vi "Scope_5782_6channel_IQ_PID.vi"() -> ()   [LabVIEW 2018]
uses:
  FPGA/DataMode.ctl
  <vilib>/Analysis/4window.llb/windowTd.ctl
  Host/Scope/controls/power_spectrum_unit.ctl
  Host/Scope5782/Scope/controls/5782_trigger_type.ctl
  Host/Scope/controls/Data_calc_mode.ctl
  Host/Scope/controls/Data_display_mode.ctl
  Host/Scope/controls/Graph_references.ctl
  Host/Scope/controls/graph_controls.ctl
  Host/Scope/controls/Channel_select_2fpga.ctl
  <vilib>/userdefined/High Color/nirio_resource_hc.ctl
  Host/Scope/controls/All FP controls.ctl
  Host/Scope/controls/Output scale.ctl
  Host/Communication/Driver/RemoteConnection/RemoteReferences.ctl
  Host/FpgaRef/FpgaRef5761/ClockSource_5761.ctl
  Host/INI files/Settings file IQ PID/SettingsFileIQpid.lvclass
  C:/PXIe/InProgress/source/Host/INI files/Settings file base/SettingsFile.lvclass
  Host/Communication/Driver/RemoteConnection/RemoteConnection.lvclass
  Host/Scope/Scope5782_six_channel/Scope5782_six_channel.lvclass
  C:/PXIe/InProgress/source/Host/Scope/ScopeBase/ScopeBase.lvclass
  Host/Scope/ScopeBase/ScopeBase.lvclass/ScopeBase.ctl
  Host/INI files/Settings file base/Save event.ctl
  FPGA/fpga_settings.ctl
  Host/Scope/Scope5782_six_channel/Scope5782_six_channel.lvclass/Scope5782_six_channel.ctl
  Host/Scope/controls/ScopeMode.ctl
  Host/FpgaRef/FpgaRef5761/FpgaRef5761.lvclass
  C:/PXIe/InProgress/source/Host/FpgaRef/FpgaRefBase/FpgaRefBase.lvclass
  Host/FpgaRef/FpgaRef5782/FpgaRef5782.lvclass
  Host/Communication/global_stop.vi
  <vilib>/FPGAPlugInAG/PXIe-7975R/niLvFpga_Open_PXIe-7975R.vi
  <vilib>/rvi/interface/common/dynamic/niFpgaDynamicAddResources.vi
  Host/Communication/response.ctl
  Host/Communication/driver_status.ctl
  <vilib>/rvi/interface/nirviOpenFPGA/nirviOpenFPGA.xnode
  FPGA Bitfiles/FPGAmain_5782_IQ_PID_PtIU9Q++q2U.lvbitx
  FPGA Bitfiles/FPGAmain_5761_zuew0qNtRjU.lvbitx
  <vilib>/rvi/FXPMathLib/FxpInterpret/XNode/nifxpmath_Interpret.xnode
  Host/Communication/Driver/TcpServerDriver/TcpServerDriver.lvclass
  Host/Scope/ScopeBase/ScopeBase.lvclass
  Host/INI files/Settings file base/SettingsFile.lvclass
  Host/FpgaRef/FpgaRefBase/FpgaRefBase.lvclass
  <vilib>/Analysis/NI_AALPro.lvlib
panel:
  out "All FP controls":T1
  in  "Show buffers":bool
  out "Adaptive FF graph":dbl[][](graph)
  in  "Tab Control":T2(tab)
  in  "Feedback I":bool caption="I Feedback"
  in  "Ki*T AM":fxp<+/-,32,4> caption="Ki*T"
  in  "Kd/T AM":fxp<+/-,32,4> caption="Kd/T"
  in  "Kp AM":fxp<+/-,32,4> caption="Kp"
  in  "Feedback delay":u32
  in  "Trigger delay":u32
  in  "Acquire samples":u32
  in  "Kp Q":fxp<+/-,32,4> caption="Kp"
  in  "Kd/T  Q":fxp<+/-,32,4> caption="Kd/T"
  in  "Ki*T Q":fxp<+/-,32,4> caption="Ki*T"
  in  "Feedback Q":bool caption="Q Feedback"
  in  "Host scale 5761":T3 caption="Host scale"
  in  "Input scale 5761":T3 caption="Input scale"
  in  "Host scale":T3
  in  "Input scale":T3
  in  "Output scale":T3
  in  "ch2 DC offset":dbl caption="DC offset\nChannel 2"
  in  "ch3 DC offset":dbl caption="DC offset\nChannel 3"
  in  "ch0 DC offset 2":dbl caption="DC offset\nChannel 0"
  in  "ch1 DC offset 2":dbl caption="DC offset\nChannel 1"
  in  "ch0 DC offset":dbl caption="DC offset\nChannel 0"
  in  "ch1 DC offset":dbl caption="DC offset\nChannel 1"
  in  "Setpoint":path
  in  "Beam":path
  in  "Feed forward":path
  in  "show setpoint":bool
  in  "show beam":bool
  in  "show feedforward":bool
  in  "Setpoint enabled":bool
  in  "Beam/FF enabled":bool
  in  "IIR filter cutoff fequency [MHz]":dbl min=0.0 max=10000.0
  in  "Save FF to file":bool
  in  "Clear buffers":bool
  in  "Samples to skip":i32 min=0 max=400000
  in  "Adaptation factor [0-1]":dbl min=0.0 max=1.0
  in  "LP filter cutoff fequency [MHz]":dbl min=0.0 max=10000.0
  in  "Adaptive FF enabled":bool
  in  "Read buffers":bool
  in  "Virtual cavity":bool
  in  "Cavity model":bool
  in  "w12":dbl format="%#_12g"
  in  "R1":dbl
  in  "w1":dbl
  in  "Q1":dbl
  in  "K1":dbl
  in  "S":dbl=0.001 min=0.001 max=1000.0 format="%#_12g"
  in  "Input delay 5785":u32
  in  "Input delay 5761":u32
  in  "5761 resource":T4="PXI2Slot11"
  in  "5782 resource":T4="PXI2Slot18"
  in  "High speed transfer to host":bool=TRUE
  in  "Output enabled":bool=TRUE
  in  "Output delay delta":dbl(slide) scale=0.0..6.0
  in  "Output delay":dbl(slide) scale=0.0..6.0
  in  "Output mixer fequency [MHz]":dbl
  in  "Trigger":T5
  in  "Mode":T6
  in  "Mixer freq [MHz]":dbl
  in  "Unwrap phase":bool
  in  "#bins":i32=1 min=1 max=16
  in  "Unit":T7
  in  "Window":T8=1 items=["Rectangle"=0, "Hanning"=1, "Hamming"=2, "Blackman-Harris"=3, "Exact Blackman"=4, "Blackman"=5, "Flat Top"=6, "4 Term B-Harris "=7, "7 Term B-Harris"=8, "Low Sidelobe"=9, "Blackman Nuttall"=11, "Triangle"=30, "Bartlett-Hanning"=31, "Bohman"=32, "Parzen"=33, "Welch"=34, "Kaiser"=60, "Dolph-Chebyshev"=61, "Gaussian"=62]
  in  "Chart length":i32=400000
  in  "Trigmode":enum32{"Triggered", "Continuous"}(radio)
  in  "Reference for phase":T9
  in  "Graph_refs":T10
  out "Lower chart":dbl[][](graph)
  out "Upper chart":dbl[][](graph)
  out "Lower graph":i16[][](graph)
  in  "Buffer":T12
  in  "Display":T13
  out "stop 2":bool
  in  "Zoom freq X":bool
  in  "Zoom freq Y":bool
  in  "Zoom time Y":bool
  in  "Zoom time X":bool
  in  "Samples per 5782 record":i32
  in  "Phase offset (deg)":dbl
  in  "Fequency [MHz]":dbl format="%#_8g"
  out "freqdata":cluster{"f0":dbl, "df":dbl, "magnitude":dbl[]}[](graph)
  out "Upper graph":i16[][](graph)
  in  "Rumode":bool
  in  "Singleshot":bool
  out "error IO":errorcluster
  in  "stop":bool
  # "FPGA setup"
  # "ns"
  # "Output delay"
  # "Auto Zoom"
  # "FFT"
  # "Auto Zoom"
  # "Delays"
  # "5785"
  # "5761"
  # "5782"
  # "V"
  # "V"
  # "5761"
  # "V"
  # "V"
  # "V"
  # "V"
  # "Simulated data"
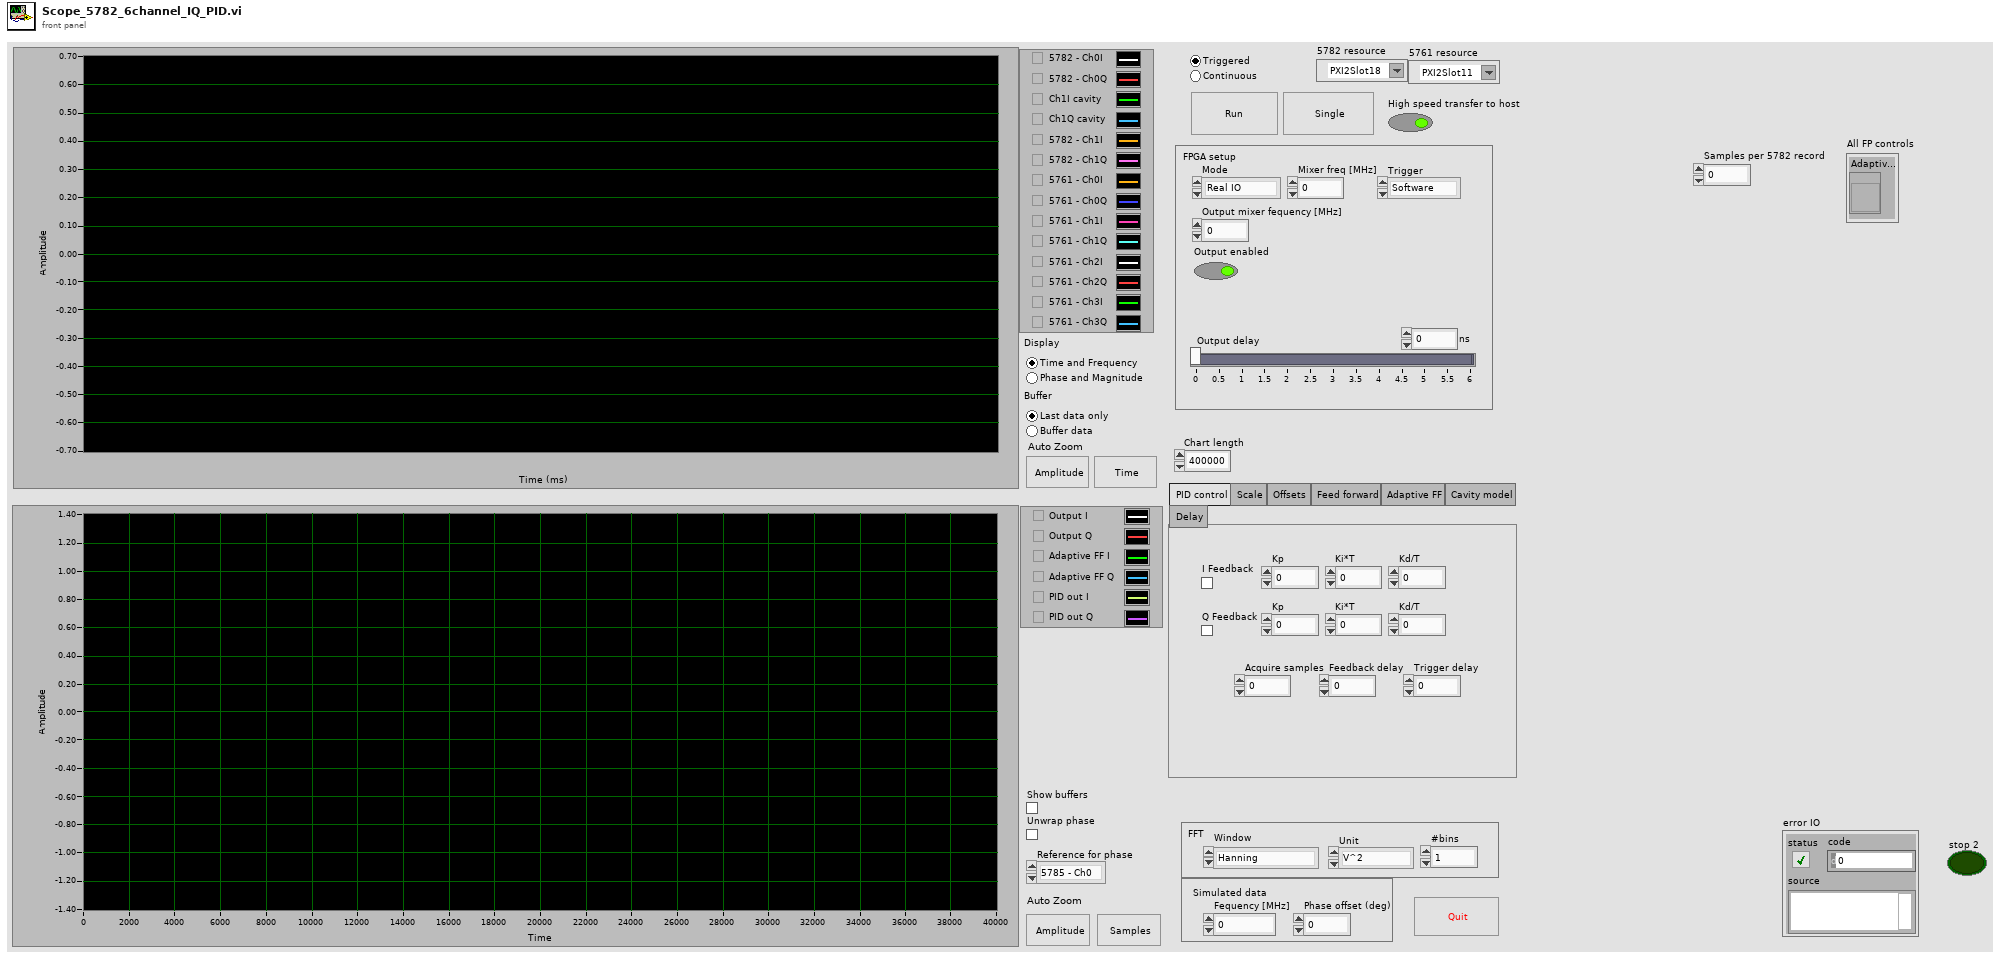
[diagram p1: front panel]
types:
  T1 = typedef "All FP controls.ctl" = cluster{"Adaptive FF enabled":refnum<vi>, "LP filter cutoff fequency [MHz]":refnum<vi>, "Adaptation factor [0-1]":refnum<vi>, "Samples to skip":refnum<vi>, "ch1 DC offset":refnum<vi>, "ch0 DC offset":refnum<vi>, "ch1 DC offset 2":refnum<vi>, "ch0 DC offset 2":refnum<vi>, "ch3 DC offset":refnum<vi>, "ch2 DC offset":refnum<vi>, "Feedback Q":refnum<vi>, "Ki*T Q":refnum<vi>, "Kd/T  Q":refnum<vi>, "Kp Q":refnum<vi>, "Acquire samples":refnum<vi>, "Trigger delay":refnum<vi>, "Feedback delay":refnum<vi>, "Kp AM":refnum<vi>, "Kd/T AM":refnum<vi>, "Ki*T AM":refnum<vi>, "Feedback I":refnum<vi>, "#bins":refnum<vi>, "Window":refnum<vi>, "Unit":refnum<vi>, "Input delay 5761":refnum<vi>, "Input delay 5785":refnum<vi>, "S":refnum<vi>, "K1":refnum<vi>, "Q1":refnum<vi>, "R1":refnum<vi>, "w12":refnum<vi>, "Cavity model":refnum<vi>, "w1":refnum<vi>, "Mode":refnum<vi>, "Trigger":refnum<vi>, "Output mixer fequency [MHz]":refnum<vi>, "Output delay":refnum<vi>, "Mixer freq [MHz]":refnum<vi>, "Triggered":refnum<vi>, "High speed transfer to host":refnum<vi>, "Continuous":refnum<vi>, "Output scale":refnum<vi>, "Host scale":refnum<vi>, "Input scale":refnum<vi>, "IIR filter cutoff fequency [MHz]":refnum<vi>, "Host scale 5761":refnum<vi>, "Virtual cavity":refnum<vi>, "Input scale 5761":refnum<vi>}
  T2 = enum32{"PID control", "Scale", "Offsets", "Feed forward", "Adaptive FF", "Cavity model", "Delay"}
  T3 = typedef "Output scale.ctl" = enum16{"x1", "x2", "x4", "x8", "x16", "x32"}
  T4 = typedef "nirio_resource_hc.ctl" = tag
  T5 = typedef "5782_trigger_type.ctl" = enum16{"Software", "Trigger input"}
  T6 = typedef "DataMode.ctl" = enum16{"Real IO", "Simulated"}
  T7 = typedef "power_spectrum_unit.ctl" = enum16{"V^2", "V", "dBV"}
  T8 = typedef "NI_AALPro.lvlib/windowTd.ctl" = u32
  T9 = typedef "Channel_select_2fpga.ctl" = enum16{"5785 - Ch0", "5785 - Ch1 cavity", "5785 - Ch1", "5761 - Ch0", "5761 - Ch1", "5761 - Ch2", "5761 - Ch3"}
  T10 = typedef "Graph_references.ctl" = cluster{"upper":T11, "lower":T11, "Freq graph":refnum<vi>, "Adaptive FF graph":refnum<vi>}
  T11 = typedef "graph_controls.ctl" = cluster{"Graph":refnum<vi>, "Time btn":refnum<vi>, "Amplitude btn":refnum<vi>, "Chart":refnum<vi>}
  T12 = typedef "Data_display_mode.ctl" = enum32{"Last data only", "Buffer data"}
  T13 = typedef "Data_calc_mode.ctl" = enum32{"Time and Frequency", "Phase and Magnitude"}
  T14 = typedef "ClockSource_5761.ctl" = enum8{"Internal Clock PLL Off", "Internal Clock PLL On (CLK_IN)", "External Clock (CLK_IN)", "Internal Clock PLL On (IoModSyncClk)", "External Clock (IoModSyncClk)"}
  T15 = typedef "RemoteConnection.lvclass/RemoteReferences.ctl" = cluster{"a":refnum<vi>, "b":refnum<vi>, "fm":refnum<vi>, "Output delay":refnum<vi>, "Output delay delta":refnum<vi>}
  T16 = typedef "response.ctl" = cluster{"driver status":T17, "Sender":string, "Type":i32, "Variant":variant}
  T17 = typedef "driver_status.ctl" = enum16{"Normal", "Startup", "Connection lost", "Reconnected", "Timeout", "Idle", "Busy"}
  T18 = typedef "message_queue.ctl" = refnum<queue>
  T19 = enum8{"Internal Clock PLL Off", "Internal Clock PLL On (REF IN)", "External Clock (CLK_IN)", "Internal Clock PLL On (IoModSyncClk)"}
  T20 = typedef "INI Save Event.ctl" = refnum<user-event>
  T21 = typedef "Save event.ctl" = cluster{"Automatic":bool, "Save":bool}
  T22 = typedef "fpga_settings.ctl" = enum16{"Feedback Enable", "New FIR coeffs", "FIR shift", "Enable filter", "Set Downsample", "Downsample", "CIC Gain", "Record length", "Trigger samples", "Quiet time", "a_am", "b_am", "Use fixed delay", "fixed sin_fi", "fixed cos_fi", "Ki*Tau", "Kp", "Kd_Tau", "Fi_start", "Fi_delta", "DC_offs 0", "DC_offs 1", "DC_offs 2", "DC_offs 3", "Ki*Tau am", "Kp am", "Kd_Tau am", "Feedback AM", "Trigger delay", "Feedback delay", "Setpoint enable", "Beam enable", "Samples to acquire", "Cavity Enable", "Cavity C1", "Cavity C2", "Cavity C3", "Cavity C4", "Cavity C5", "Input delay", "Ki*Tau Q", "Kp Q", "Kd_Tau Q", "Adaptive FF enable", "Feedforward a0", "Feedforward b0", "FF src adress", "FF dest adress", "Output scale", "Input scale", "Host scale", "FF_IIR b0", "FF_IIR b1", "FF_IIR b2", "FF_IIR-a1", "FF_IIR-a2", "Enable HW trigger", "Virtual cavity"}
  T23 = typedef "ScopeMode.ctl" = enum16{"Stopped", "Single", "Running", "Continuous"}
  T24 = enum8{"Enabled", "Disabled", "Disabled and Grayed Out"}
  T25 = typedef "Feedforward.ctl" = cluster{"Beam I":dbl[], "Beam Q":dbl[], "Feedforward I":dbl[], "Feedforward Q":dbl[], "Setpoint I":dbl[], "Setpoint Q":dbl[]}
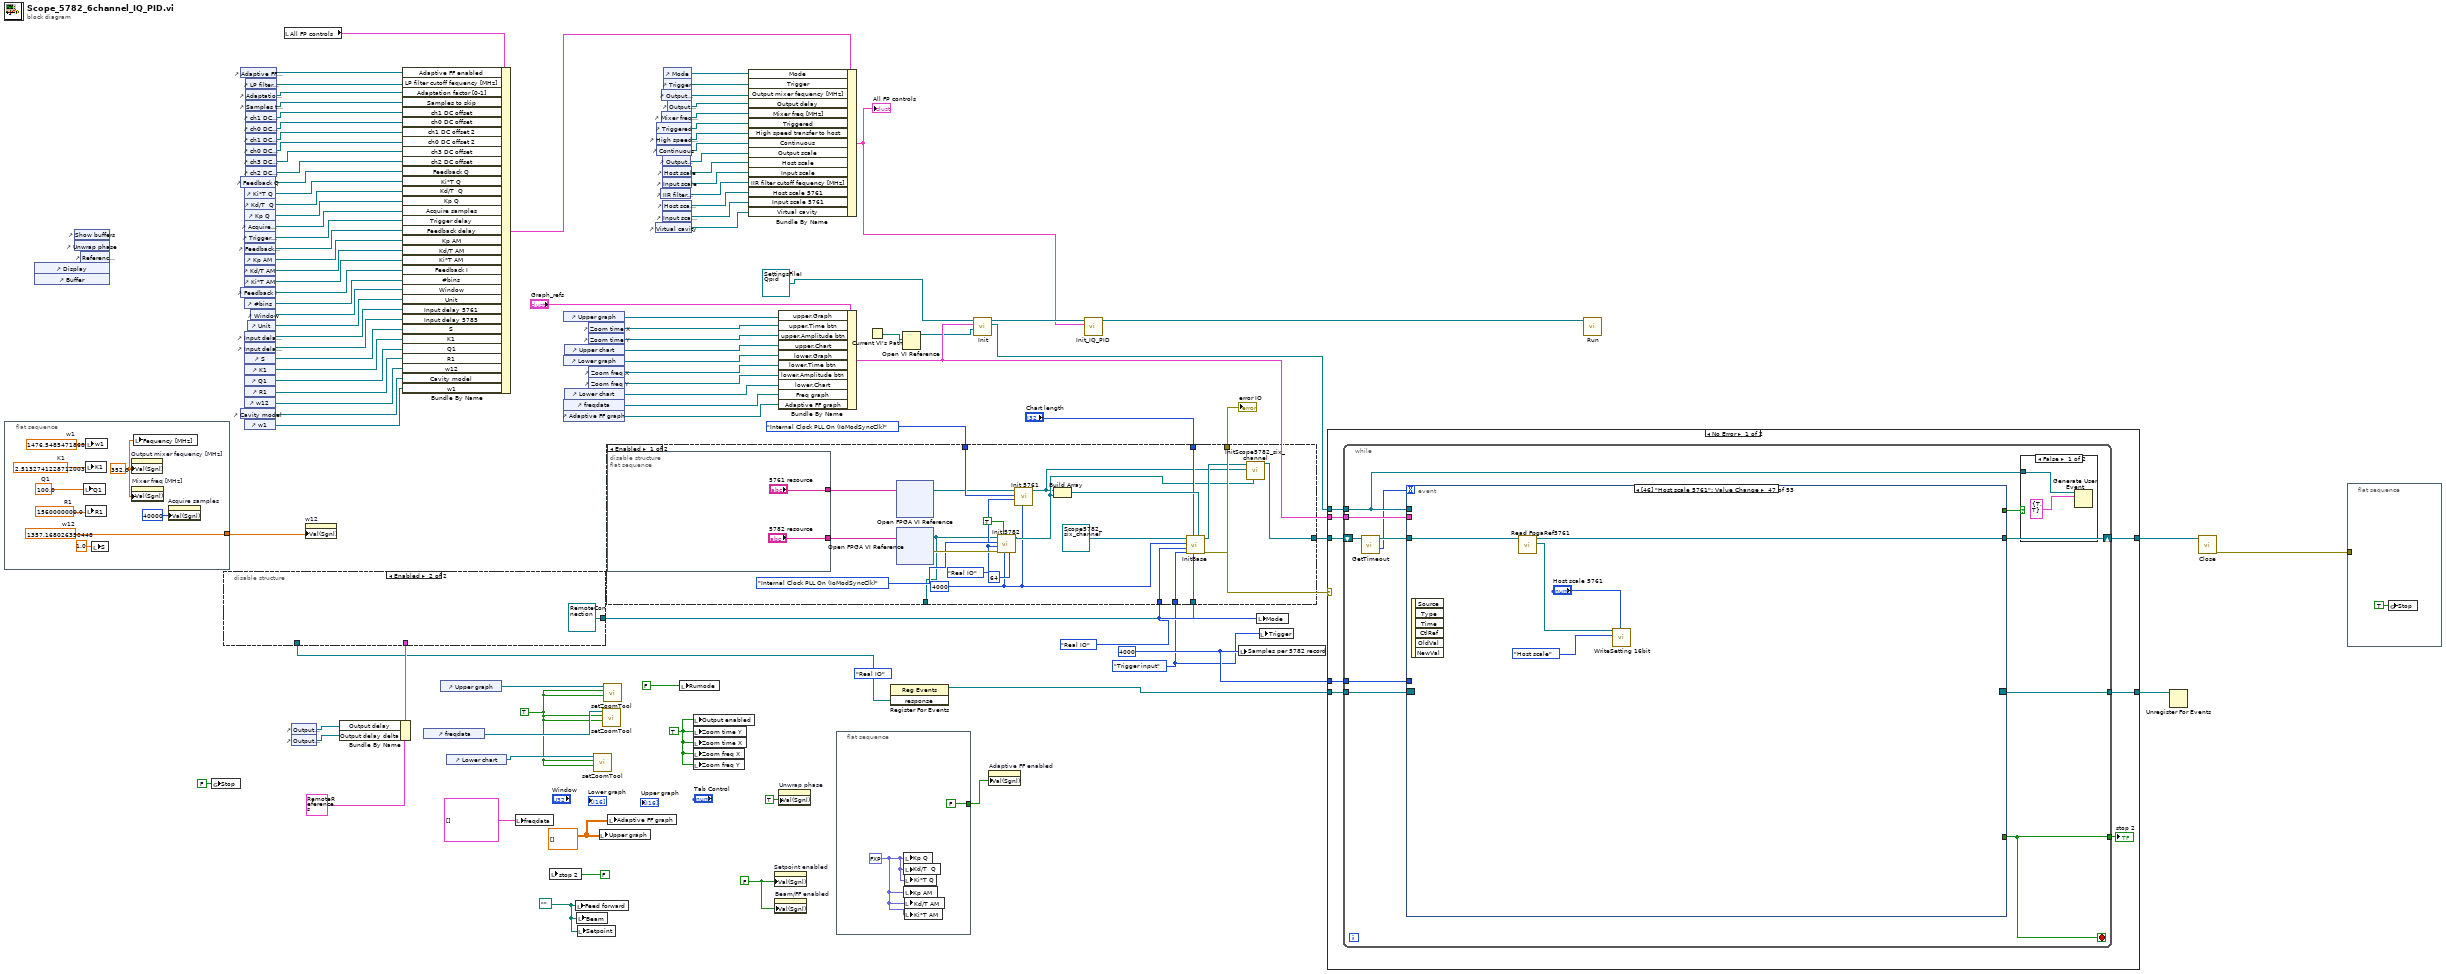
[diagram p0: block diagram]
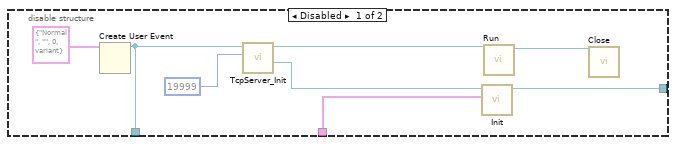
[diagram p3: hidden frame]
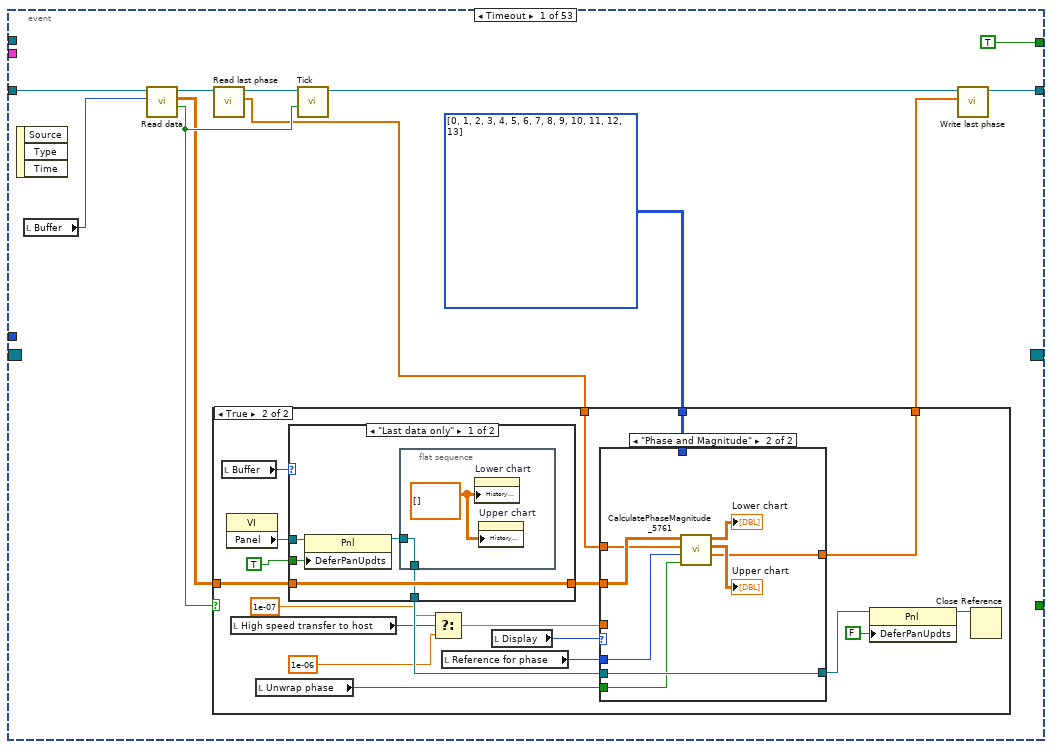
[diagram p5: hidden frame]
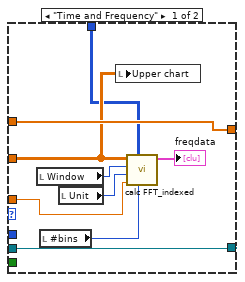
[diagram p8: hidden frame]
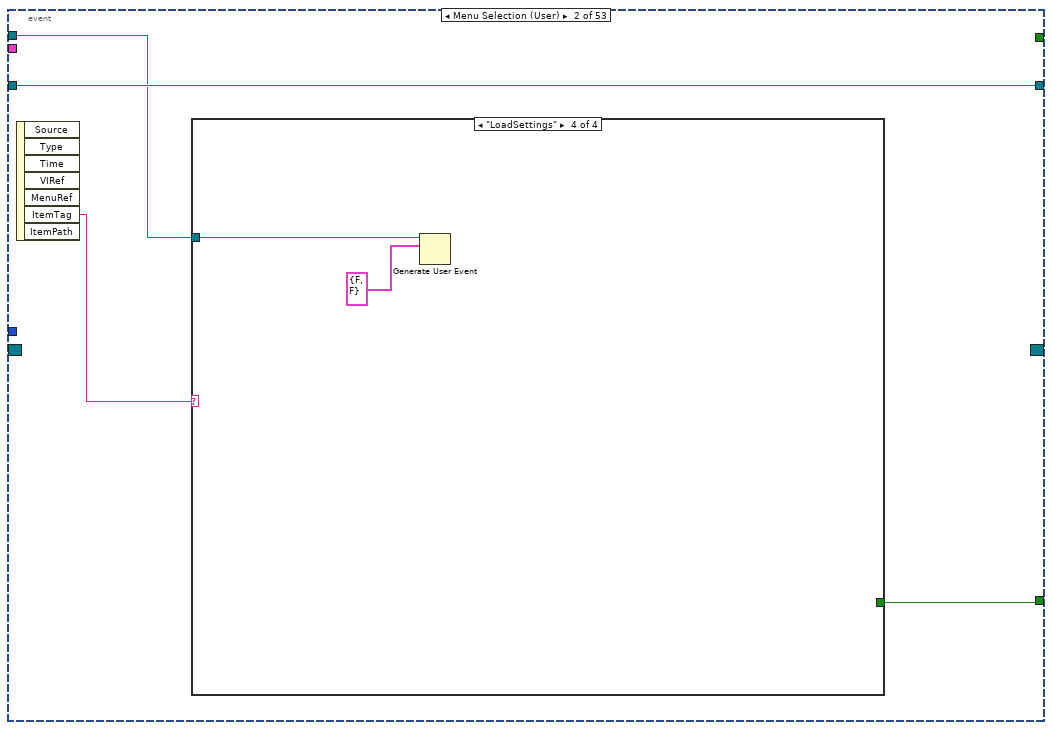
[diagram p9: hidden frame]
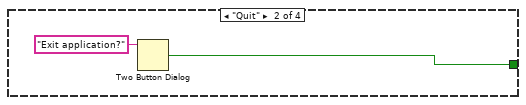
[diagram p11: hidden frame]
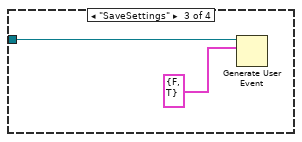
[diagram p12: hidden frame]
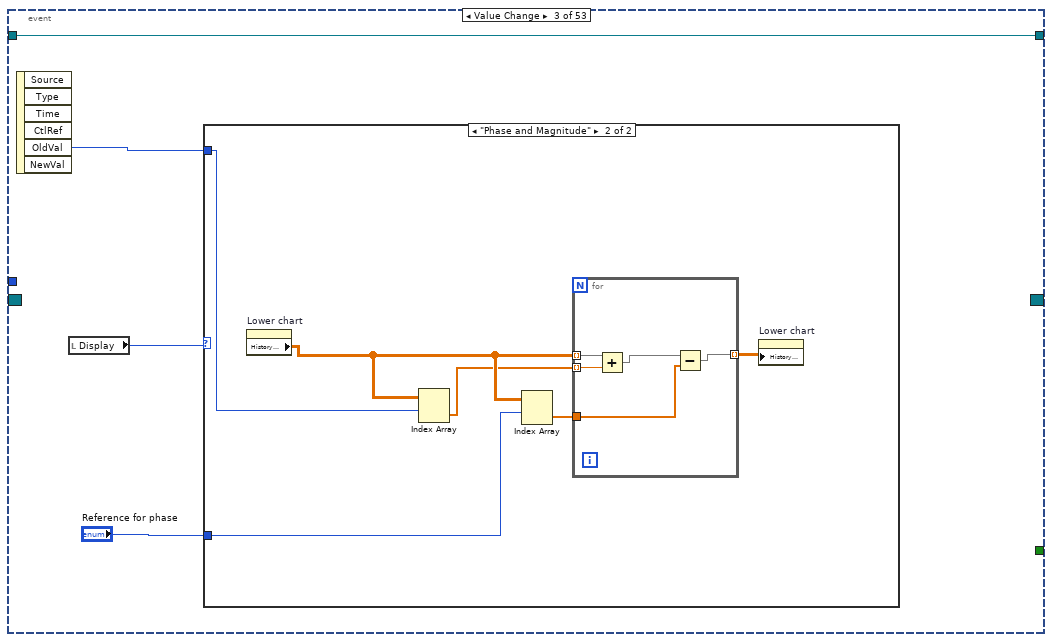
[diagram p13: hidden frame]
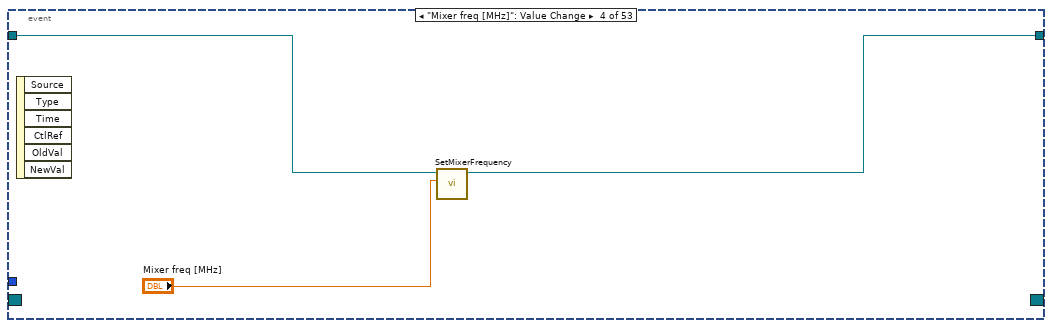
[diagram p15: hidden frame]
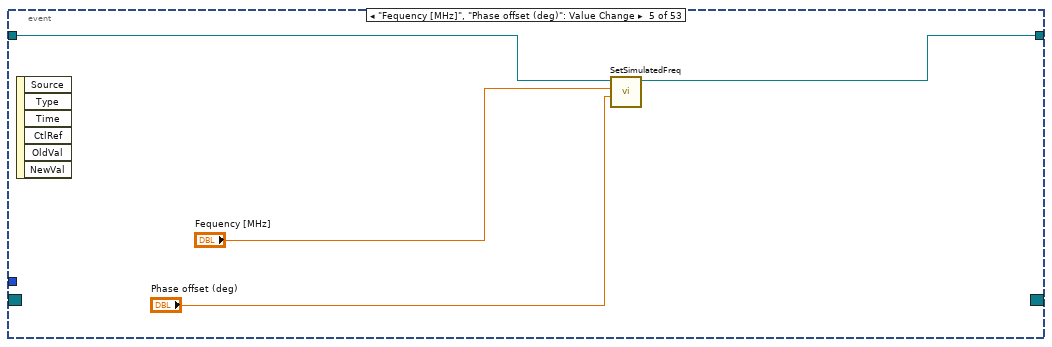
[diagram p16: hidden frame]
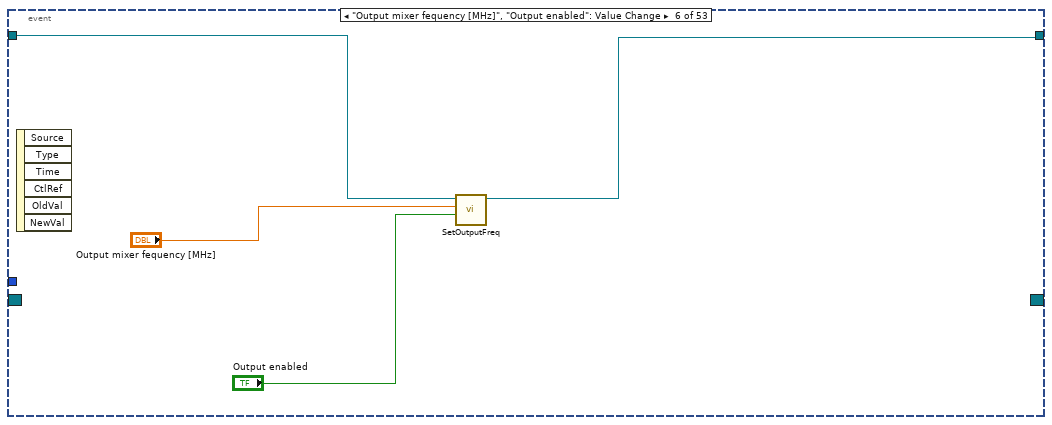
[diagram p17: hidden frame]
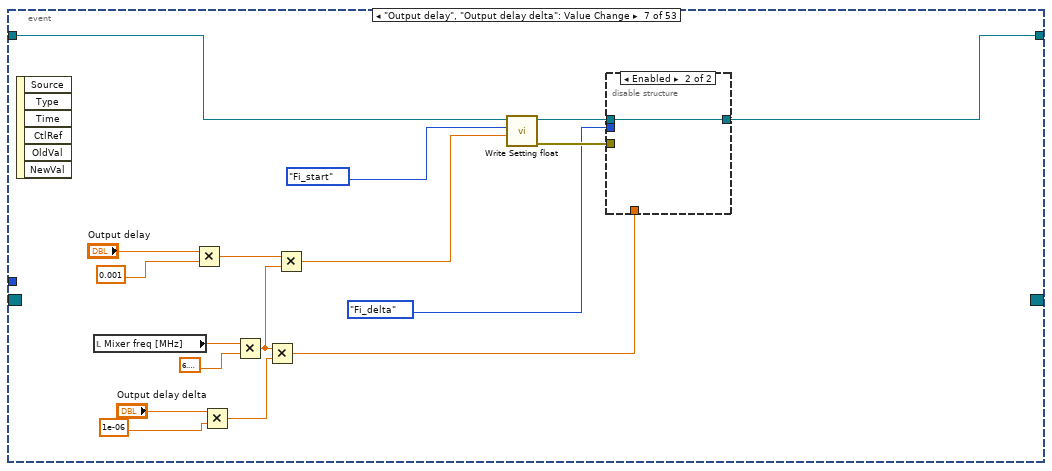
[diagram p18: hidden frame]
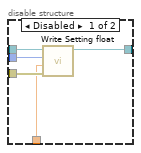
[diagram p19: hidden frame]
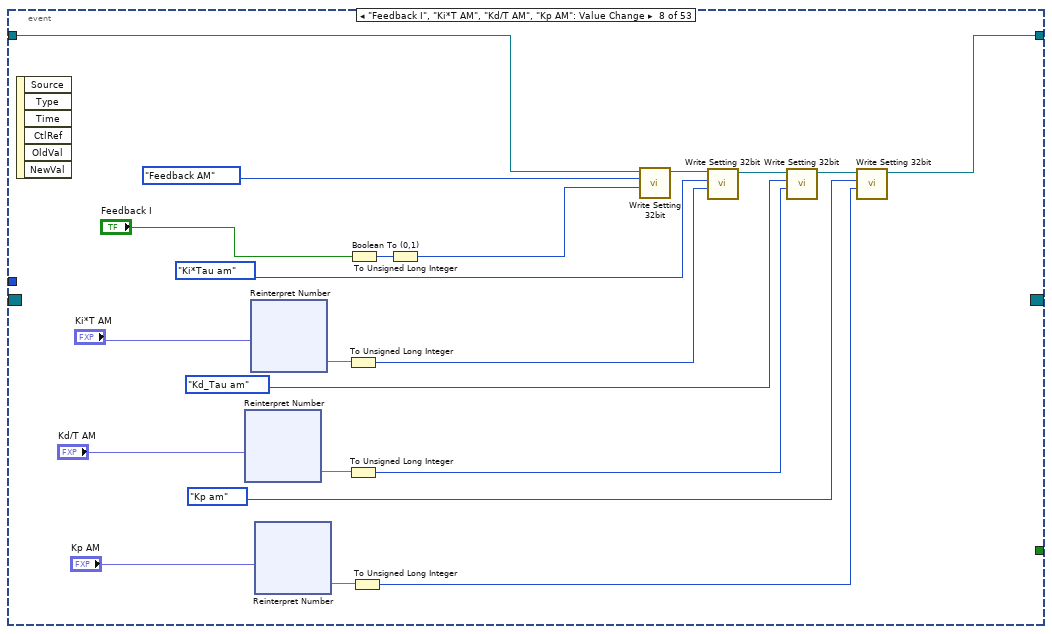
[diagram p20: hidden frame]
diagram:
  (unwired) DataMode."Real IO" ("Mode")
  w70 = DataMode."Real IO" ("Mode")
  w72 = path "" ("Feed forward")
  w73 = FALSE ("Value (Signaling)")
  w69 = 5782_trigger_type."Trigger input" ("Trigger")
  w80 = TRUE ("Zoom  X")
  w76 = TRUE ("Rumode")
  w75 = 4000 ("Samples to aqcuire")
  w61 = dbl[][] [] ("Timedata")
  n1 = flat-sequence {
    tunnel: [w104] -> w9
    frame #0 {
      w102 = 352.0 ("Value (Signaling)")
      w106 = 2.5132741228712003  # K1
      w105 = 100.0  # Q1
      w107 = 1476.54854718683  # w1
      w108 = 1560000000.0  # R1
      w104 = 1357.168026350448  # w12
      n2 = local write "Q1"(w105) -> ()
      n3 = local write "w1"(w107) -> ()
      n4 = local write "K1"(w106) -> ()
      n5 = local write "R1"(w108) -> ()
      n6 = local write "S"(1.0 ("S")) -> ()
      n7 = property on="Output mixer fequency [MHz]" class="DigNum (strict)"("Val(Sgnl)"=w102) -> ()  [unwired: 2 in, 2 out]
      n8 = property on="Mixer freq [MHz]" class="DigNum (strict)"("Val(Sgnl)"=w102) -> ()  [unwired: 2 in, 2 out]
      n9 = local write "Fequency [MHz]"(w102) -> ()
      n10 = property on="Acquire samples" class="DigNum (strict)"("Val(Sgnl)"=u32 40000 ("Value (Signaling)")) -> ()  [unwired: 2 in, 2 out]
    }
  }
  n11 = control-ref of="Display"() -> ()  [unwired: 1 out]
  n12 = control-ref of="Buffer"() -> ()  [unwired: 1 out]
  n13 = control-ref of="Show buffers"() -> ()  [unwired: 1 out]
  n14 = control-ref of="Unwrap phase"() -> ()  [unwired: 1 out]
  n15 = control-ref of="Reference for phase"() -> ()  [unwired: 1 out]
  n16 = global write "global_stop.vi" "Stop"(FALSE ("Stop")) -> ()
  n17 = control-ref of="Feedback Q"() -> (w49:refnum<vi>)
  n18 = control-ref of="Feedback I"() -> (w39:refnum<vi>)
  n19 = control-ref of="Cavity model"() -> (w28:refnum<vi>)
  n20 = control-ref of="Adaptive FF enabled"() -> (w59:refnum<vi>)
  n21 = control-ref of="Ki*T Q"() -> (w48:refnum<vi>)
  n22 = control-ref of="Kd/T  Q"() -> (w47:refnum<vi>)
  n23 = control-ref of="Kp Q"() -> (w46:refnum<vi>)
  n24 = control-ref of="Acquire samples"() -> (w45:refnum<vi>)
  n25 = control-ref of="Trigger delay"() -> (w44:refnum<vi>)
  n26 = control-ref of="Feedback delay"() -> (w43:refnum<vi>)
  n27 = control-ref of="Kp AM"() -> (w42:refnum<vi>)
  n28 = control-ref of="Kd/T AM"() -> (w41:refnum<vi>)
  n29 = control-ref of="Ki*T AM"() -> (w40:refnum<vi>)
  n30 = control-ref of="#bins"() -> (w38:refnum<vi>)
  n31 = control-ref of="Input delay 5761"() -> (w35:refnum<vi>)
  n32 = control-ref of="Input delay 5785"() -> (w34:refnum<vi>)
  n33 = control-ref of="S"() -> (w33:refnum<vi>)
  n34 = control-ref of="K1"() -> (w32:refnum<vi>)
  n35 = control-ref of="Q1"() -> (w31:refnum<vi>)
  n36 = control-ref of="R1"() -> (w30:refnum<vi>)
  n37 = control-ref of="w12"() -> (w29:refnum<vi>)
  n38 = control-ref of="w1"() -> (w27:refnum<vi>)
  n39 = control-ref of="LP filter cutoff fequency [MHz]"() -> (w58:refnum<vi>)
  n40 = control-ref of="Adaptation factor [0-1]"() -> (w57:refnum<vi>)
  n41 = control-ref of="Samples to skip"() -> (w56:refnum<vi>)
  n42 = control-ref of="ch1 DC offset"() -> (w55:refnum<vi>)
  n43 = control-ref of="ch0 DC offset"() -> (w54:refnum<vi>)
  n44 = control-ref of="ch1 DC offset 2"() -> (w53:refnum<vi>)
  n45 = control-ref of="ch0 DC offset 2"() -> (w52:refnum<vi>)
  n46 = control-ref of="ch3 DC offset"() -> (w51:refnum<vi>)
  n47 = control-ref of="ch2 DC offset"() -> (w50:refnum<vi>)
  n48 = control-ref of="Unit"() -> (w36:refnum<vi>)
  n49 = control-ref of="Window"() -> (w37:refnum<vi>)
  n50 = local read "All FP controls"() -> (w60:T1)
  n51 = control-ref of="Output delay"() -> (w79:refnum<vi>)
  n52 = control-ref of="Output delay delta"() -> (w78:refnum<vi>)
  n53 = property on="w12" class="DigNum (strict)"("Val(Sgnl)"=w9) -> ()  [unwired: 2 in, 2 out]
  n54 = Bundle By Name(cluster=T15 {"a"=refnum, "b"=refnum, "fm"=refnum, "Output delay"=refnum, "Output delay delta"=refnum} ("refs"), "Output delay"=w79, "Output delay delta"=w78) -> (w85:T15)
  n55 = disable-structure shown="Enabled" {
    disable-tunnel: w85 -> [w117 _]
    disable-tunnel: [w112 _] -> w82
    disable-tunnel: [w110 refnum<class "RemoteConnection.lvclass"> refnum ("RemoteConnection")] -> w68
    frame Disabled {
      n56 = Create User Event(user event datatype=T16 {"driver status"=enum."Normal", "Sender"="", "Type"=0, "Variant"=variant} ("response")) -> (user event=w112:refnum<user-event>)  [unwired: 1 in, 1 out]
      n57 = call "TcpServer_Init.vi"("local port"=u16 19999, "response event"=w112) -> ("Message queue"=w116:T18, "TcpServerDriver"=w114:refnum<class "TcpServerDriver.lvclass">)  [unwired: 8 in]
      n58 = call "Init.vi"("refs"=w117, "server queue"=w116) -> ("RemoteConnection"=w110:refnum<class "RemoteConnection.lvclass">)  [unwired: 9 in]
      n59 = call-dynamic "Run.vi"("BaseDriver in"=w114) -> ("BaseDriver out"=w115:refnum<class "TcpServerDriver.lvclass">)  [unwired: 9 in, 1 out]
      n60 = call-dynamic "Close.vi"("BaseDriver in"=w115) -> ()  [unwired: 9 in, 2 out]
    }
    frame Enabled {
    }
  }
  n61 = Bundle By Name(cluster=w60, "Adaptive FF enabled"=w59, "LP filter cutoff fequency [MHz]"=w58, "Adaptation factor [0-1]"=w57, "Samples to skip"=w56, "ch1 DC offset"=w55, "ch0 DC offset"=w54, "ch1 DC offset 2"=w53, "ch0 DC offset 2"=w52, "ch3 DC offset"=w51, "ch2 DC offset"=w50, "Feedback Q"=w49, "Ki*T Q"=w48, "Kd/T  Q"=w47, "Kp Q"=w46, "Acquire samples"=w45, "Trigger delay"=w44, "Feedback delay"=w43, "Kp AM"=w42, "Kd/T AM"=w41, "Ki*T AM"=w40, "Feedback I"=w39, "#bins"=w38, "Window"=w37, "Unit"=w36, "Input delay 5761"=w35, "Input delay 5785"=w34, "S"=w33, "K1"=w32, "Q1"=w31, "R1"=w30, "w12"=w29, "Cavity model"=w28, "w1"=w27) -> (w26:T1)
  n62 = control-ref of="freqdata"() -> (w96:refnum<vi>)
  n63 = control-ref of="Upper graph"() -> (w97:refnum<vi>)
  n64 = control-ref of="Lower chart"() -> (w81:refnum<vi>)
  n65 = local write "freqdata"(cluster{"f0":dbl, "df":dbl, "magnitude":dbl[]}[] [] ("freqdata")) -> ()
  n66 = local write "stop 2"(FALSE ("stop 2")) -> ()
  n67 = control-ref of="Upper graph"() -> (w94:refnum<vi>)
  n68 = control-ref of="Lower graph"() -> (w90:refnum<vi>)
  n69 = control-ref of="freqdata"() -> (w86:refnum<vi>)
  n70 = control-ref of="Adaptive FF graph"() -> (w62:refnum<vi>)
  n71 = control-ref of="Upper chart"() -> (w91:refnum<vi>)
  n72 = control-ref of="Lower chart"() -> (w87:refnum<vi>)
  n73 = local write "Feed forward"(w72) -> ()
  n74 = local write "Beam"(w72) -> ()
  n75 = local write "Setpoint"(w72) -> ()
  n76 = control-ref of="Zoom time X"() -> (w93:refnum<vi>)
  n77 = control-ref of="Zoom time Y"() -> (w92:refnum<vi>)
  n78 = control-ref of="Zoom freq X"() -> (w89:refnum<vi>)
  n79 = control-ref of="Zoom freq Y"() -> (w88:refnum<vi>)
  n80 = call "setZoomTool.vi"("Zoom Y"=w80, "Zoom  X"=w80, "reference"=w81) -> ()  [unwired: 9 in]
  n81 = local write "Upper graph"(w61) -> ()
  n82 = call "setZoomTool.vi"("Zoom Y"=w80, "Zoom  X"=w80, "reference"=w96) -> ()  [unwired: 9 in]
  n83 = call "setZoomTool.vi"("Zoom Y"=w80, "Zoom  X"=w80, "reference"=w97) -> ()  [unwired: 9 in]
  n84 = disable-structure shown="Enabled" {
    disable-tunnel: ClockSource_5761."Internal Clock PLL On (IoModSyncClk)" ("Clock Source") -> [w140 _]
    disable-tunnel: w70 -> [w136 _]
    disable-tunnel: w69 -> [w135 _]
    disable-tunnel: w68 -> [w134 _]
    disable-tunnel: "Chart length" -> [w133 _]
    disable-tunnel: [w132 _] -> w7
    disable-tunnel: [w128 _] -> w63
    disable-tunnel: [w119 _] -> _
    frame Enabled {
      w120 = u16 4000 ("Samples to aqcuire")
      w123 = DataMode."Real IO" ("Mode")
      n85 = flat-sequence {
        tunnel: ["5761 resource"] -> w138
        tunnel: ["5782 resource"] -> w137
        frame #0 {
        }
      }
      n86 = xnode "Open FPGA VI Reference"("resource name"=w138) -> ("FPGA VI Reference Out"=w125:refnum<k20>)  [unwired: 1 in, 1 out]
      n87 = xnode "Open FPGA VI Reference"("resource name"=w137) -> ("FPGA VI Reference Out"=w119:refnum<k20>, "error out"=w130:errorcluster)  [unwired: 1 in]
      n88 = call "Init 5782.vi"("User Data 1"=u8 64, "Record length"=w120, "Use 1Mhz clock"=TRUE, "error in (no error)"=w130, "Mode"=w123, "Clock Source"=T19."Internal Clock PLL On (IoModSyncClk)", "FPGA ref"=w119) -> ("FpgaRef5782 Out"=w127:refnum<class "FpgaRef5782.lvclass">)  [unwired: 3 in, 1 out]
      n89 = call "Init 5761.vi"("Record length"=w120, "Mode"=w123, "Clock Source"=w140, "FPGA ref"=w125) -> ("FpgaRef5761 out"=w126:refnum<class "FpgaRef5761.lvclass">)  [unwired: 6 in, 1 out]
      n90 = Build Array(w126, w127) -> (w139:refnum<class "FpgaRefBase.lvclass">[])
      n91 = call "InitBase.vi"("FPGA refs"=w139, "RemoteConnection"=w134, "Chart length"=w133, "Trigger"=w135, "data mode"=w136, "Samples Per Trigger"=w120, "ScopeBase in"=refnum<class "Scope5782_six_channel.lvclass"> refnum ("Scope5761")) -> ("error out"=w132:errorcluster, "ScopeBase out"=w129:refnum<class "Scope5782_six_channel.lvclass">)  [unwired: 3 in]
      n92 = call "InitScope5782_six_channel.vi"("FpgaRef5782"=w127, "FpgaRef5761"=w126, "Scope5785_six_channel"=w129) -> ("Scope5785_six_channel out"=w128:refnum<class "Scope5782_six_channel.lvclass">)  [unwired: 7 in, 1 out]
    }
    frame Disabled {
    }
  }
  "error IO" <- w7
  n93 = local write "Adaptive FF graph"(w61) -> ()
  n94 = control-ref of="Virtual cavity"() -> (w1:refnum<vi>)
  n95 = control-ref of="Triggered"() -> (w20:refnum<vi>)
  n96 = control-ref of="High speed transfer to host"() -> (w19:refnum<vi>)
  n97 = control-ref of="Continuous"() -> (w18:refnum<vi>)
  n98 = control-ref of="IIR filter cutoff fequency [MHz]"() -> (w4:refnum<vi>)
  n99 = control-ref of="Output mixer fequency [MHz]"() -> (w23:refnum<vi>)
  n100 = control-ref of="Mixer freq [MHz]"() -> (w21:refnum<vi>)
  n101 = control-ref of="Output scale"() -> (w8:refnum<vi>)
  n102 = control-ref of="Host scale"() -> (w6:refnum<vi>)
  n103 = control-ref of="Input scale"() -> (w5:refnum<vi>)
  n104 = control-ref of="Host scale 5761"() -> (w3:refnum<vi>)
  n105 = control-ref of="Input scale 5761"() -> (w2:refnum<vi>)
  n106 = control-ref of="Mode"() -> (w25:refnum<vi>)
  n107 = control-ref of="Trigger"() -> (w24:refnum<vi>)
  n108 = control-ref of="Output delay"() -> (w22:refnum<vi>)
  n109 = local write "Rumode"(FALSE ("Rumode")) -> ()
  n110 = local write "Output enabled"(w76) -> ()
  n111 = local write "Zoom time Y"(w76) -> ()
  n112 = local write "Zoom time X"(w76) -> ()
  n113 = local write "Zoom freq X"(w76) -> ()
  n114 = local write "Zoom freq Y"(w76) -> ()
  n115 = Bundle By Name(cluster=w26, "Mode"=w25, "Trigger"=w24, "Output mixer fequency [MHz]"=w23, "Output delay"=w22, "Mixer freq [MHz]"=w21, "Triggered"=w20, "High speed transfer to host"=w19, "Continuous"=w18, "Output scale"=w8, "Host scale"=w6, "Input scale"=w5, "IIR filter cutoff fequency [MHz]"=w4, "Host scale 5761"=w3, "Input scale 5761"=w2, "Virtual cavity"=w1) -> (w10:T1)
  "All FP controls" <- w10
  n116 = property on="Setpoint enabled" class="Bool (strict)"("Val(Sgnl)"=w73) -> ()  [unwired: 2 in, 2 out]
  n117 = property on="Beam/FF enabled" class="Bool (strict)"("Val(Sgnl)"=w73) -> ()  [unwired: 2 in, 2 out]
  n118 = Bundle By Name(cluster="Graph_refs", "upper.Graph"=w94, "upper.Time btn"=w93, "upper.Amplitude btn"=w92, "upper.Chart"=w91, "lower.Graph"=w90, "lower.Time btn"=w89, "lower.Amplitude btn"=w88, "lower.Chart"=w87, "Freq graph"=w86, "Adaptive FF graph"=w62) -> (w17:T10)
  n119 = property on="Unwrap phase" class="Bool (strict)"("Val(Sgnl)"=TRUE ("Value (Signaling)")) -> ()  [unwired: 2 in, 2 out]
  n120 = flat-sequence {
    tunnel: [FALSE] -> w64
    frame #0 {
      w143 = fxp<+/-,32,4> 0.0 ("Kp")
      n121 = local write "Kp Q"(w143) -> ()
      n122 = local write "Kd/T  Q"(w143) -> ()
      n123 = local write "Kp AM"(w143) -> ()
      n124 = local write "Ki*T Q"(w143) -> ()
      n125 = local write "Kd/T AM"(w143) -> ()
      n126 = local write "Ki*T AM"(w143) -> ()
    }
  }
  n127 = Current VI's Path() -> (path=w16:path)
  n128 = register-events(w82) -> (reference out=w100:refnum<event-registration>)  [unwired: 2 in, 1 out]
  n129 = Open VI Reference(vi path=w16) -> (vi reference=w15:refnum<vi>)  [unwired: 5 in, 1 out]
  n130 = call "Init.vi"("vi reference"=w15, "Graph_refs"=w17, "SettingsFile in"=refnum<class "SettingsFileIQpid.lvclass"> refnum ("SettingsFileIQpid.lvclass")) -> ("Save event"=w13:T20, "SettingsFile out"=w12:refnum<class "SettingsFileIQpid.lvclass">)  [unwired: 6 in, 1 out]
  n131 = property on="Adaptive FF enabled" class="Bool (strict)"("Val(Sgnl)"=w64) -> ()  [unwired: 2 in, 2 out]
  n132 = call "Init_IQ_PID.vi"("All FP controls"=w10, "SettingsFileIQpid in"=w12) -> ("SettingsFileIQpid out"=w11:refnum<class "SettingsFileIQpid.lvclass">)  [unwired: 8 in, 1 out]
  n133 = local write "Samples per 5782 record"(w75) -> ()
  n134 = local write "Mode"(w70) -> ()
  n135 = local write "Trigger"(w69) -> ()
  n136 = case shown="No Error" w7 {
    tunnel: w63 -> [w152 w640]
    tunnel: [w151 w640] -> w66
    tunnel: w100 -> [w150 w639]
    tunnel: [w149 w639] -> w99
    tunnel: w17 -> [w147 _]
    tunnel: w75 -> [w146 _]
    tunnel: w13 -> [w145 _]
    frame No Error {
      n137 = while {
        shift-right: [w156] -> w151
        shift-left: w152 -> [w163]
        tunnel: w150 -> [w161]
        tunnel: [w160] -> w149
        tunnel: [w159] -> w148
        tunnel: w147 -> [w158]
        tunnel: w146 -> [w157]
        tunnel: w145 -> [w154]
        stop <- w159 stop-if-true
        n138 = call "GetTimeout.vi"("ScopeBase in"=w163) -> ("Time left"=w153:i32, "ScopeBase out"=w162:refnum<class "Scope5782_six_channel.lvclass">)  [unwired: 8 in, 1 out]
        n139 = event shown="[46] \"Host scale 5761\": Value Change" {
          selector: w161 -> [_ _ _ _ _ _ _ _ _ _ _ _ _ _ _ _ _ _ _ _ _ _ _ _ _ _ _ _ _ _ _ _ _ _ _ _ _ _ _ _ _ _ _ _ _ _ _ _ _ _ _ _ _]
          dyn-events: [_ _ _ _ _ _ _ _ _ _ _ _ _ _ _ _ _ _ _ _ _ _ _ _ _ _ _ _ _ _ _ _ _ _ _ _ _ _ _ _ _ _ _ _ _ _ _ _ _ _ _ _ _] -> w160
          timeout: w153 -> [_ _ _ _ _ _ _ _ _ _ _ _ _ _ _ _ _ _ _ _ _ _ _ _ _ _ _ _ _ _ _ _ _ _ _ _ _ _ _ _ _ _ _ _ _ _ _ _ _ _ _ _ _]
          tunnel: [_ w225 _ _ _ _ _ _ _ _ _ _ _ _ _ _ _ _ _ _ _ _ _ _ _ _ _ _ _ _ _ _ "stop" _ _ _ _ _ _ _ _ _ _ _ _ _ _ _ _ _ _ _ _] -> w159
          tunnel: w162 -> [w177 w227 w237 w251 w253 w259 w267 w292 w313 w326 w337 w342 w347 w352 w357 w365 w368 w372 w385 w396 w411 w412 w421 w431 w440 w446 w450 w455 w472 w473 w478 w487 w488 w495 w506 w511 w518 w527 w534 w544 w548 w557 w562 w567 w572 w575 w581 w587 w594 w599 w605 w620 w630]
          tunnel: [w170 w227 w237 w249 w252 w256 w260 w291 w312 w325 w336 w341 w346 w351 w356 w359 w367 w373 w384 w397 w410 w413 w420 w430 w439 w444 w448 w451 w470 w474 w477 w487 w488 w495 w506 w511 w518 w527 w530 w543 w546 w556 w561 w566 w571 w574 w580 w586 w593 w598 w613 w620 w638] -> w156
          tunnel: w158 -> [_ _ _ _ _ _ _ _ _ _ _ _ _ _ _ _ _ _ _ _ _ _ _ _ _ _ _ _ _ _ _ _ _ _ _ _ _ w524 _ _ _ _ _ _ _ _ _ _ _ _ _ _ _]
          tunnel: w157 -> [_ _ _ _ _ _ _ _ _ _ _ _ _ _ _ _ _ _ _ _ _ _ _ _ _ _ _ w467 _ _ _ _ _ _ _ _ _ _ _ _ _ _ _ _ _ _ _ _ _ _ _ _ _]
          tunnel: w154 -> [_ w224 _ _ _ _ _ _ _ _ _ _ _ _ _ _ _ _ _ _ _ _ _ _ _ _ _ _ _ _ _ _ _ _ _ _ _ _ _ _ _ _ _ _ _ _ _ _ _ _ _ _ _]
          tunnel: [TRUE _ _ _ _ _ _ _ _ _ _ _ _ _ _ _ _ _ _ _ _ _ _ _ _ _ _ _ _ _ _ _ _ _ _ _ _ _ _ _ _ _ _ _ _ _ _ _ _ _ _ _ _] -> w155
          event Timeout {
            n140 = event-data() -> ()  [unwired: 1 in, 3 out]
            n141 = local read "Buffer"() -> (w176:T12)
            n142 = call-dynamic "Read data.vi"("Buffer mode"=w176, "Scope5785_six_channel"=w177) -> ("Any read?"=w173:bool, "Data"=w168:dbl[][], "Scope5785_six_channel out"=w175:refnum<class "Scope5782_six_channel.lvclass">)  [unwired: 6 in, 1 out]
            n143 = call "Read last phase.vi"("ScopeBase in"=w175) -> ("last phase"=w172:dbl[], "ScopeBase out"=w174:refnum<class "Scope5782_six_channel.lvclass">)  [unwired: 8 in, 1 out]
            n144 = case shown="True" w173 {
              tunnel: w168 -> [_ w194]
              tunnel: w172 -> [w178 w186]
              tunnel: [w178 w185] -> w169
              tunnel: i32[][] [[0, 1], [2, 3], [4, 5], [6, 7], [8, 9], [10, 11], [12, 13]] ("IQ indexes") -> [_ w179]
              frame False {
              }
              frame True {
                n145 = local read "Buffer"() -> (w196:T12)
                n146 = property class="VI"() -> ("Panel"=w189:refnum<vi>)  [unwired: 2 in, 2 out]
                n147 = local read "High speed transfer to host"() -> (w184:bool)
                n148 = local read "Unwrap phase"() -> (w180:bool)
                n149 = case shown="\"Last data only\"" w196 {
                  tunnel: w194 -> [w202 w206]
                  tunnel: [w202 w206] -> w195
                  tunnel: w189 -> [w201 w205]
                  tunnel: TRUE ("Defer Panel Updates") -> [w199 _]
                  tunnel: [w198 w205] -> w187
                  frame "Last data only" {
                    n150 = property class="Pnl"(reference=w201, "DeferPanUpdts"=w199) -> (reference out=w200:refnum<vi>)  [unwired: 1 in, 1 out]
                    n151 = flat-sequence {
                      tunnel: w200 -> [w203]
                      tunnel: [w203] -> w198
                      frame #0 {
                        w204 = dbl[][] [] ("History Data")
                        n152 = property on="Lower chart" class="WFChart (strict)"("History Data"=w204) -> ()  [unwired: 2 in, 2 out]
                        n153 = property on="Upper chart" class="WFChart (strict)"("History Data"=w204) -> ()  [unwired: 2 in, 2 out]
                      }
                    }
                  }
                  frame "Buffer data" {
                  }
                }
                n154 = Select(t=1e-07 ("dt"), s=w184, f=1e-06 ("dt")) -> (s? t:f=w181:dbl)
                n155 = local read "Reference for phase"() -> (w193:T9)
                n156 = local read "Display"() -> (w197:T13)
                n157 = case shown="\"Phase and Magnitude\"" w197 {
                  tunnel: w195 -> [w208 w223]
                  tunnel: w193 -> [_ w220]
                  tunnel: [w212 w219] -> w191
                  tunnel: w187 -> [w212 w219]
                  tunnel: w186 -> [w210 w218]
                  tunnel: [w210 w217] -> w185
                  tunnel: w181 -> [w209 _]
                  tunnel: w180 -> [_ w216]
                  tunnel: w179 -> [w207 _]
                  frame "Time and Frequency" {
                    n158 = local read "Window"() -> (w213:T8)
                    n159 = local read "#bins"() -> (w211:i32)
                    n160 = local read "Unit"() -> (w214:T7)
                    n161 = local write "Upper chart"(w208) -> ()
                    n162 = call "calc FFT_indexed.vi"("#bins"=w211, "IQ indexes"=w207, "dt"=w209, "Unit"=w214, "Window"=w213, "data"=w208) -> ("Power Spectrum / PSD"=→"freqdata":cluster{"f0":dbl, "df":dbl, "magnitude":dbl[]}[])  [unwired: 5 in]
                  }
                  frame "Phase and Magnitude" {
                    n163 = call "CalculatePhaseMagnitude_5761.vi"("unwrap phase"=w216, "phase reference channel"=w220, "previous phase"=w218, "data"=w223) -> ("last phase"=w217:dbl[], "Magnitude"=→"Upper chart":dbl[][], "Phase"=→"Lower chart":dbl[][])  [unwired: 5 in]
                  }
                }
                n164 = property class="Pnl"(reference=w191, "DeferPanUpdts"=FALSE ("Defer Panel Updates")) -> (reference out=w190:refnum<vi>)  [unwired: 1 in, 1 out]
                n165 = Close Reference(reference=w190) -> ()  [unwired: 1 in, 1 out]
              }
            }
            n166 = call "Tick.vi"("Any elements read?"=w173, "ScopeBase in"=w174) -> ("ScopeBase out"=w171:refnum<class "Scope5782_six_channel.lvclass">)  [unwired: 8 in, 1 out]
            n167 = call "Write last phase.vi"("last phase"=w169, "ScopeBase in"=w171) -> ("ScopeBase out"=w170:refnum<class "Scope5782_six_channel.lvclass">)  [unwired: 8 in, 1 out]
          }
          event Menu Selection (User) {
            n168 = event-data() -> ("ItemTag"=w226:string)  [unwired: 1 in, 6 out]
            n169 = case shown="\"LoadSettings\"" w226 {
              tunnel: [_ w228 _ _] -> w225
              tunnel: w224 -> [_ _ w231 w233]
              frame "False", Default {
              }
              frame "Quit" {
                n170 = Two Button Dialog(message="Exit application?") -> (T button?=w228:bool)  [unwired: 2 in]
              }
              frame "SaveSettings" {
                n171 = Generate User Event(user event=w231, event data cluster=T21 {"Automatic"=FALSE, "Save"=TRUE} ("event data")) -> ()  [unwired: 2 in, 2 out]
              }
              frame "LoadSettings" {
                n172 = Generate User Event(user event=w233, event data cluster=T21 {"Automatic"=FALSE, "Save"=FALSE} ("event data")) -> ()  [unwired: 2 in, 2 out]
              }
            }
          }
          event Value Change {
            n173 = event-data() -> ("OldVal"=w234:T9)  [unwired: 1 in, 5 out]
            n174 = local read "Display"() -> (w235:T13)
            n175 = case shown="\"Phase and Magnitude\"" w235 {
              tunnel: "Reference for phase" -> [_ w242]
              tunnel: w234 -> [_ w240]
              frame "Time and Frequency", Default {
              }
              frame "Phase and Magnitude" {
                n176 = property on="Lower chart" class="WFChart (strict)"() -> ("History Data"=w241:dbl[][])  [unwired: 2 in, 2 out]
                n177 = Index Array(array=w241, index (row)=w240) -> (element=w239:dbl[])  [unwired: 1 in]
                n178 = Index Array(array=w241, index (row)=w242) -> (element=w243:dbl[])  [unwired: 1 in]
                n179 = for {
                  tunnel: w241 -> [w246] mode=indexing
                  tunnel: w243 -> [w248]
                  tunnel: [w247] -> w238 mode=indexing
                  tunnel: w239 -> [w245] mode=indexing
                  n180 = Add(x=w246, y=w245) -> (x+y=w244:dbl[])
                  n181 = Subtract(x=w244, y=w248) -> (x-y=w247:dbl[])
                }
                n182 = property on="Lower chart" class="WFChart (strict)"("History Data"=w238) -> ()  [unwired: 2 in, 2 out]
              }
            }
          }
          event "Mixer freq [MHz]": Value Change {
            n183 = event-data() -> ()  [unwired: 1 in, 6 out]
            n184 = call-dynamic "SetMixerFrequency.vi"("Mixer freq [MHz]"="Mixer freq [MHz]", "Scope5785_six_channel"=w251) -> ("Scope5785_six_channel Out"=w249:refnum<class "Scope5782_six_channel.lvclass">)  [unwired: 8 in, 1 out]
          }
          event "Fequency [MHz]", "Phase offset (deg)": Value Change {
            n185 = event-data() -> ()  [unwired: 1 in, 6 out]
            n186 = call-dynamic "SetSimulatedFreq.vi"("Phase offset (deg)"="Phase offset (deg)", "Mixer freq [MHz]"="Fequency [MHz]", "Scope5785_six_channel"=w253) -> ("Scope5785_six_channel out"=w252:refnum<class "Scope5782_six_channel.lvclass">)  [unwired: 7 in, 1 out]
          }
          event "Output mixer fequency [MHz]", "Output enabled": Value Change {
            n187 = event-data() -> ()  [unwired: 1 in, 6 out]
            n188 = call "SetOutputFreq.vi"("Output enabled"="Output enabled", "Output mixer fequency [MHz]"="Output mixer fequency [MHz]", "Scope5785_six_channel"=w259) -> ("Scope5785_six_channel out"=w256:refnum<class "Scope5782_six_channel.lvclass">)  [unwired: 7 in, 1 out]
          }
          event "Output delay", "Output delay delta": Value Change {
            n189 = event-data() -> ()  [unwired: 1 in, 6 out]
            n190 = local read "Mixer freq [MHz]"() -> (w270:dbl)
            n191 = Multiply(x="Output delay", y=0.001) -> (x*y=w271:dbl)
            n192 = Multiply(x="Output delay delta", y=1e-06) -> (x*y=w273:dbl)
            n193 = Multiply(x=w270, y=6.283185307179586) -> (x*y=w268:dbl)
            n194 = Multiply(x=w268, y=w273) -> (x*y=w262:dbl)
            n195 = Multiply(x=w271, y=w268) -> (x*y=w265:dbl)
            n196 = call "Write Setting float.vi"("value"=w265, "FPGA Setting"=fpga_settings."Fi_start", "ScopeBase in"=w267) -> ("error out"=w263:errorcluster, "ScopeBase out"=w264:refnum<class "Scope5782_six_channel.lvclass">)  [unwired: 7 in]
            n197 = disable-structure shown="Enabled" {
              disable-tunnel: w264 -> [w281 w282]
              disable-tunnel: w263 -> [w280 _]
              disable-tunnel: w262 -> [w279 _]
              disable-tunnel: fpga_settings."Fi_delta" ("FPGA Setting") -> [w278 _]
              disable-tunnel: [w277 w282] -> w260
              frame Disabled {
                n198 = call "Write Setting float.vi"("error in (no error)"=w280, "value"=w279, "FPGA Setting"=w278, "ScopeBase in"=w281) -> ("ScopeBase out"=w277:refnum<class "Scope5782_six_channel.lvclass">)  [unwired: 6 in, 1 out]
              }
              frame Enabled {
              }
            }
          }
          event "Feedback I", "Ki*T AM", "Kd/T AM", "Kp AM": Value Change {
            n199 = event-data() -> ()  [unwired: 1 in, 6 out]
            n200 = xnode "Reinterpret Number"("x"="Kd/T AM") -> ("y"=w301:fxp<+,32,32>)
            n201 = xnode "Reinterpret Number"("x"="Ki*T AM") -> ("y"=w300:fxp<+,32,32>)
            n202 = xnode "Reinterpret Number"("x"="Kp AM") -> ("y"=w302:fxp<+,32,32>)
            n203 = To Unsigned Long Integer(number=w300) -> (unsigned 32bit integer=w285:u32)
            n204 = To Unsigned Long Integer(number=w301) -> (unsigned 32bit integer=w284:u32)
            n205 = Boolean To (0,1)(Boolean="Feedback I") -> (0, 1=w303:i16)
            n206 = To Unsigned Long Integer(number=w302) -> (unsigned 32bit integer=w283:u32)
            n207 = To Unsigned Long Integer(number=w303) -> (unsigned 32bit integer=w289:u32)
            n208 = call "Write Setting 32bit.vi"("value"=w289, "FPGA Setting"=fpga_settings."Feedback AM", "ScopeBase in"=w292) -> ("ScopeBase out"=w295:refnum<class "Scope5782_six_channel.lvclass">)  [unwired: 7 in, 1 out]
            n209 = call "Write Setting 32bit.vi"("value"=w285, "FPGA Setting"=fpga_settings."Ki*Tau am", "ScopeBase in"=w295) -> ("ScopeBase out"=w294:refnum<class "Scope5782_six_channel.lvclass">)  [unwired: 7 in, 1 out]
            n210 = call "Write Setting 32bit.vi"("value"=w284, "FPGA Setting"=fpga_settings."Kd_Tau am", "ScopeBase in"=w294) -> ("ScopeBase out"=w293:refnum<class "Scope5782_six_channel.lvclass">)  [unwired: 7 in, 1 out]
            n211 = call "Write Setting 32bit.vi"("value"=w283, "FPGA Setting"=fpga_settings."Kp am", "ScopeBase in"=w293) -> ("ScopeBase out"=w291:refnum<class "Scope5782_six_channel.lvclass">)  [unwired: 7 in, 1 out]
          }
          event "Kp Q", "Kd/T  Q", "Ki*T Q", "Feedback Q": Value Change {
            n212 = event-data() -> ()  [unwired: 1 in, 6 out]
            n213 = xnode "Reinterpret Number"("x"="Kd/T  Q") -> ("y"=w322:fxp<+,32,32>)
            n214 = xnode "Reinterpret Number"("x"="Ki*T Q") -> ("y"=w321:fxp<+,32,32>)
            n215 = xnode "Reinterpret Number"("x"="Kp Q") -> ("y"=w323:fxp<+,32,32>)
            n216 = To Unsigned Long Integer(number=w321) -> (unsigned 32bit integer=w306:u32)
            n217 = To Unsigned Long Integer(number=w322) -> (unsigned 32bit integer=w305:u32)
            n218 = Boolean To (0,1)(Boolean="Feedback Q") -> (0, 1=w324:i16)
            n219 = To Unsigned Long Integer(number=w323) -> (unsigned 32bit integer=w304:u32)
            n220 = To Unsigned Long Integer(number=w324) -> (unsigned 32bit integer=w310:u32)
            n221 = call "Write Setting 32bit.vi"("value"=w310, "FPGA Setting"=fpga_settings."Feedback Enable", "ScopeBase in"=w313) -> ("ScopeBase out"=w316:refnum<class "Scope5782_six_channel.lvclass">)  [unwired: 7 in, 1 out]
            n222 = call "Write Setting 32bit.vi"("value"=w306, "FPGA Setting"=fpga_settings."Ki*Tau Q", "ScopeBase in"=w316) -> ("ScopeBase out"=w315:refnum<class "Scope5782_six_channel.lvclass">)  [unwired: 7 in, 1 out]
            n223 = call "Write Setting 32bit.vi"("value"=w305, "FPGA Setting"=fpga_settings."Kd_Tau Q", "ScopeBase in"=w315) -> ("ScopeBase out"=w314:refnum<class "Scope5782_six_channel.lvclass">)  [unwired: 7 in, 1 out]
            n224 = call "Write Setting 32bit.vi"("value"=w304, "FPGA Setting"=fpga_settings."Kp Q", "ScopeBase in"=w314) -> ("ScopeBase out"=w312:refnum<class "Scope5782_six_channel.lvclass">)  [unwired: 7 in, 1 out]
          }
          event "w12", "R1", "w1", "Q1", "K1", "S": Value Change {
            n225 = event-data() -> ()  [unwired: 1 in, 6 out]
            n226 = call "CavityConstanstToFIFO.vi"("w12"="w12", "R1"="R1", "w1"="w1", "Q1"="Q1", "K1"="K1", "S"="S") -> ("FIFO array"=w327:u64[])  [unwired: 9 in]
            n227 = call "Write Setting Array.vi"("Data"=w327, "ScopeBase in"=w326) -> ("ScopeBase out"=w325:refnum<class "Scope5782_six_channel.lvclass">)  [unwired: 8 in, 1 out]
          }
          event "ch0 DC offset": Value Change {
            n228 = event-data() -> ()  [unwired: 1 in, 6 out]
            n229 = call "Read FpgaRef5782.vi"("Scope5785_six_channel"=w337) -> ("FpgaRef5782.lvclass"=w338:refnum<class "FpgaRef5782.lvclass">, "Scope5785_six_channel Out"=w336:refnum<class "Scope5782_six_channel.lvclass">)  [unwired: 8 in, 1 out]
            n230 = call "SetDcOffset.vi"("FPGA Setting"=fpga_settings."DC_offs 0", "DC offset"="ch0 DC offset", "FpgaRef5782 in"=w338) -> ()  [unwired: 7 in, 2 out]
          }
          event "ch0 DC offset 2": Value Change {
            n231 = event-data() -> ()  [unwired: 1 in, 6 out]
            n232 = call "Read FpgaRef5761.vi"("Scope5785_six_channel"=w342) -> ("FpgaRef5761.lvclass"=w343:refnum<class "FpgaRef5761.lvclass">, "Scope5785_six_channel Out"=w341:refnum<class "Scope5782_six_channel.lvclass">)  [unwired: 8 in, 1 out]
            n233 = call "SetDcOffset.vi"("FPGA Setting"=fpga_settings."DC_offs 0", "DC offset"="ch0 DC offset 2", "FpgaRef5761 In"=w343) -> ()  [unwired: 7 in, 2 out]
          }
          event "ch1 DC offset 2": Value Change {
            n234 = event-data() -> ()  [unwired: 1 in, 6 out]
            n235 = call "Read FpgaRef5761.vi"("Scope5785_six_channel"=w347) -> ("FpgaRef5761.lvclass"=w348:refnum<class "FpgaRef5761.lvclass">, "Scope5785_six_channel Out"=w346:refnum<class "Scope5782_six_channel.lvclass">)  [unwired: 8 in, 1 out]
            n236 = call "SetDcOffset.vi"("FPGA Setting"=fpga_settings."DC_offs 1", "DC offset"="ch1 DC offset 2", "FpgaRef5761 In"=w348) -> ()  [unwired: 7 in, 2 out]
          }
          event "ch2 DC offset": Value Change {
            n237 = event-data() -> ()  [unwired: 1 in, 6 out]
            n238 = call "Read FpgaRef5761.vi"("Scope5785_six_channel"=w352) -> ("FpgaRef5761.lvclass"=w353:refnum<class "FpgaRef5761.lvclass">, "Scope5785_six_channel Out"=w351:refnum<class "Scope5782_six_channel.lvclass">)  [unwired: 8 in, 1 out]
            n239 = call "SetDcOffset.vi"("FPGA Setting"=fpga_settings."DC_offs 2", "DC offset"="ch2 DC offset", "FpgaRef5761 In"=w353) -> ()  [unwired: 7 in, 2 out]
          }
          event "ch3 DC offset": Value Change {
            n240 = event-data() -> ()  [unwired: 1 in, 6 out]
            n241 = call "Read FpgaRef5761.vi"("Scope5785_six_channel"=w357) -> ("FpgaRef5761.lvclass"=w358:refnum<class "FpgaRef5761.lvclass">, "Scope5785_six_channel Out"=w356:refnum<class "Scope5782_six_channel.lvclass">)  [unwired: 8 in, 1 out]
            n242 = call "SetDcOffset.vi"("FPGA Setting"=fpga_settings."DC_offs 3", "DC offset"="ch3 DC offset", "FpgaRef5761 In"=w358) -> ()  [unwired: 7 in, 2 out]
          }
          event "Feedback delay", "Trigger delay": Value Change {
            n243 = event-data() -> ()  [unwired: 1 in, 6 out]
            n244 = Add(x="Feedback delay", y="Trigger delay") -> (x+y=w363:u32)
            n245 = call "Write Setting 32bit.vi"("value"=w363, "FPGA Setting"=fpga_settings."Feedback delay", "ScopeBase in"=w365) -> ("ScopeBase out"=w361:refnum<class "Scope5782_six_channel.lvclass">)  [unwired: 7 in, 1 out]
            n246 = call "Write Setting 32bit.vi"("value"="Trigger delay", "FPGA Setting"=fpga_settings."Trigger delay", "ScopeBase in"=w361) -> ("ScopeBase out"=w359:refnum<class "Scope5782_six_channel.lvclass">)  [unwired: 7 in, 1 out]
          }
          event "Acquire samples": Value Change {
            n247 = event-data() -> ()  [unwired: 1 in, 6 out]
            n248 = call "Write Setting 32bit.vi"("value"="Acquire samples", "FPGA Setting"=fpga_settings."Samples to acquire", "ScopeBase in"=w368) -> ("ScopeBase out"=w367:refnum<class "Scope5782_six_channel.lvclass">)  [unwired: 7 in, 1 out]
          }
          event "show setpoint": Value Change {
            n249 = event-data() -> ()  [unwired: 1 in, 6 out]
            n250 = call "Read Feedforward.vi"("Scope5785_six_channel"=w372) -> ("Feeforward"=w371:T25, "Scope5785_six_channel out"=w373:refnum<class "Scope5782_six_channel.lvclass">)  [unwired: 8 in, 1 out]
            n251 = Unbundle By Name(w371) -> ("Setpoint I"=w380:dbl[], "Setpoint Q"=w379:dbl[])
            n252 = Array Size(array=w380) -> (size(s)=w378:i32)
            n253 = Array Size(array=w379) -> (size(s)=w377:i32)
            n254 = Build Array(w380, w379) -> (w381:dbl[][])
            n255 = Greater Than 0?(x=w378) -> (x > 0?=w376:bool)
            n256 = Greater Than 0?(x=w377) -> (x > 0?=w375:bool)
            n257 = And(x=w376, y=w375) -> (x .and. y?=w374:bool)
            n258 = case shown="True" w374 {
              tunnel: w381 -> [_ w382]
              frame False {
              }
              frame True {
                n259 = call "ShowIQvaluesAsync.vi"("IQ data"=w382) -> ()  [unwired: 11 in]
              }
            }
          }
          event "show beam": Value Change {
            n260 = event-data() -> ()  [unwired: 1 in, 6 out]
            n261 = call "Read Feedforward.vi"("Scope5785_six_channel"=w385) -> ("Feeforward"=w383:T25, "Scope5785_six_channel out"=w384:refnum<class "Scope5782_six_channel.lvclass">)  [unwired: 8 in, 1 out]
            n262 = Unbundle By Name(w383) -> ("Beam I"=w392:dbl[], "Beam Q"=w391:dbl[])
            n263 = Array Size(array=w392) -> (size(s)=w390:i32)
            n264 = Array Size(array=w391) -> (size(s)=w389:i32)
            n265 = Build Array(w392, w391) -> (w393:dbl[][])
            n266 = Greater Than 0?(x=w390) -> (x > 0?=w388:bool)
            n267 = Greater Than 0?(x=w389) -> (x > 0?=w387:bool)
            n268 = And(x=w388, y=w387) -> (x .and. y?=w386:bool)
            n269 = case shown="True" w386 {
              tunnel: w393 -> [_ w394]
              frame False {
              }
              frame True {
                n270 = call "ShowIQvaluesAsync.vi"("IQ data"=w394) -> ()  [unwired: 11 in]
              }
            }
          }
          event "show feedforward": Value Change {
            n271 = event-data() -> ()  [unwired: 1 in, 6 out]
            n272 = call "Read Feedforward.vi"("Scope5785_six_channel"=w396) -> ("Feeforward"=w395:T25, "Scope5785_six_channel out"=w397:refnum<class "Scope5782_six_channel.lvclass">)  [unwired: 8 in, 1 out]
            n273 = Unbundle By Name(w395) -> ("Feedforward I"=w404:dbl[], "Feedforward Q"=w403:dbl[])
            n274 = Array Size(array=w404) -> (size(s)=w402:i32)
            n275 = Array Size(array=w403) -> (size(s)=w401:i32)
            n276 = Build Array(w404, w403) -> (w405:dbl[][])
            n277 = Greater Than 0?(x=w402) -> (x > 0?=w400:bool)
            n278 = Greater Than 0?(x=w401) -> (x > 0?=w399:bool)
            n279 = And(x=w400, y=w399) -> (x .and. y?=w398:bool)
            n280 = case shown="True" w398 {
              tunnel: w405 -> [_ w406]
              frame False {
              }
              frame True {
                n281 = call "ShowIQvaluesAsync.vi"("IQ data"=w406) -> ()  [unwired: 11 in]
              }
            }
          }
          event "ch1 DC offset": Value Change {
            n282 = event-data() -> ()  [unwired: 1 in, 6 out]
            n283 = call "Read FpgaRef5782.vi"("Scope5785_six_channel"=w411) -> ("FpgaRef5782.lvclass"=w409:refnum<class "FpgaRef5782.lvclass">, "Scope5785_six_channel Out"=w410:refnum<class "Scope5782_six_channel.lvclass">)  [unwired: 8 in, 1 out]
            n284 = call "SetDcOffset.vi"("FPGA Setting"=fpga_settings."DC_offs 1", "DC offset"="ch1 DC offset", "FpgaRef5782 in"=w409) -> ()  [unwired: 7 in, 2 out]
          }
          event "Setpoint enabled": Value Change {
            n285 = event-data() -> ()  [unwired: 1 in, 6 out]
            n286 = Boolean To (0,1)(Boolean="Setpoint enabled") -> (0, 1=w416:i16)
            n287 = To Word Integer(number=w416) -> (16bit integer=w418:i16)
            n288 = xnode "Reinterpret Number"("x"=w418) -> ("y"=w419:fxp<+/-,16,14>)
            n289 = xnode "Reinterpret Number"("x"=w419) -> ("y"=w415:fxp<+,16,16>)
            n290 = call "Write Setting 16bit.vi"("value"=w415, "FPGA Setting"=fpga_settings."Setpoint enable", "ScopeBase in"=w412) -> ("ScopeBase out"=w413:refnum<class "Scope5782_six_channel.lvclass">)  [unwired: 7 in, 1 out]
          }
          event "Beam/FF enabled": Value Change {
            n291 = event-data() -> ()  [unwired: 1 in, 6 out]
            n292 = Boolean To (0,1)(Boolean="Beam/FF enabled") -> (0, 1=w425:i16)
            n293 = To Word Integer(number=w425) -> (16bit integer=w426:i16)
            n294 = xnode "Reinterpret Number"("x"=w426) -> ("y"=w427:fxp<+/-,16,14>)
            n295 = xnode "Reinterpret Number"("x"=w427) -> ("y"=w422:fxp<+,16,16>)
            n296 = call "Write Setting 16bit.vi"("value"=w422, "FPGA Setting"=fpga_settings."Beam enable", "ScopeBase in"=w421) -> ("ScopeBase out"=w420:refnum<class "Scope5782_six_channel.lvclass">)  [unwired: 7 in, 1 out]
          }
          event "Cavity model": Value Change {
            n297 = event-data() -> ()  [unwired: 1 in, 6 out]
            n298 = Boolean To (0,1)(Boolean="Cavity model") -> (0, 1=w433:i16)
            n299 = To Word Integer(number=w433) -> (16bit integer=w434:i16)
            n300 = xnode "Reinterpret Number"("x"=w434) -> ("y"=w435:fxp<+/-,16,14>)
            n301 = xnode "Reinterpret Number"("x"=w435) -> ("y"=w428:fxp<+,16,16>)
            n302 = call "Write Setting 16bit.vi"("value"=w428, "FPGA Setting"=fpga_settings."Cavity Enable", "ScopeBase in"=w431) -> ("ScopeBase out"=w430:refnum<class "Scope5782_six_channel.lvclass">)  [unwired: 7 in, 1 out]
          }
          event "Virtual cavity": Value Change {
            n303 = event-data() -> ()  [unwired: 1 in, 6 out]
            n304 = Boolean To (0,1)(Boolean="Virtual cavity") -> (0, 1=w441:i16)
            n305 = To Word Integer(number=w441) -> (16bit integer=w442:i16)
            n306 = xnode "Reinterpret Number"("x"=w442) -> ("y"=w443:fxp<+/-,16,14>)
            n307 = xnode "Reinterpret Number"("x"=w443) -> ("y"=w437:fxp<+,16,16>)
            n308 = call "Write Setting 16bit.vi"("value"=w437, "FPGA Setting"=fpga_settings."Virtual cavity", "ScopeBase in"=w440) -> ("ScopeBase out"=w439:refnum<class "Scope5782_six_channel.lvclass">)  [unwired: 7 in, 1 out]
          }
          event Value Change {
            n309 = event-data() -> ()  [unwired: 1 in, 6 out]
            n310 = property on="Rumode" class="Bool (strict)"("Val(Sgnl)"=FALSE ("Value (Signaling)")) -> ()  [unwired: 2 in, 2 out]
            n311 = call-dynamic "SetMode.vi"("Mode"="Mode", "ScopeBase In"=w446) -> ("ScopeBase Out"=w444:refnum<class "Scope5782_six_channel.lvclass">)  [unwired: 8 in, 1 out]
          }
          event Value Change {
            n312 = event-data() -> ()  [unwired: 1 in, 6 out]
            n313 = call-dynamic "SetTrigger.vi"("Trigger"="Trigger", "ScopeBase In"=w450) -> ("ScopeBase Out"=w448:refnum<class "Scope5782_six_channel.lvclass">)  [unwired: 8 in, 1 out]
          }
          event "High speed transfer to host": Value Change {
            w457 = dbl[][] [] ("History Data")
            n314 = event-data() -> ()  [unwired: 1 in, 3 out]
            n315 = Multiply(x=10, y=w467) -> (x*y=w465:i32)
            n316 = Select(t=w465, s="High speed transfer to host", f=w467) -> (s? t:f=w453:i32)
            n317 = Select(t=0.0001, s="High speed transfer to host", f=0.001 ("t")) -> (s? t:f=w463:dbl)
            n318 = property on="Lower chart" class="WFChart (strict)"("History Data"=w457) -> ()  [unwired: 2 in, 2 out]
            n319 = property on="Upper chart" class="WFChart (strict)"("History Data"=w457) -> (error out=w458:errorcluster)  [unwired: 2 in, 1 out]
            n320 = Initialize Array(nan ("element"), 4 ("dimension size"), w453) -> (w460:dbl[][])
            n321 = property on="Upper chart" class="WFChart (strict)"("XScale.Multiplier"=w463) -> ()  [unwired: 2 in, 2 out]
            n322 = call-dynamic "SetRecordLength.vi"("Samples per 5782 record"=w453, "ScopeBase In"=w455) -> ("ScopeBase Out"=w454:refnum<class "Scope5782_six_channel.lvclass">)  [unwired: 8 in, 1 out]
            n323 = flat-sequence {
              tunnel: w460 -> [w469]
              tunnel: [w468] -> w456
              tunnel: w458 -> [_]
              frame #0 {
                n324 = local write "Upper chart"(w469) -> ()
                n325 = local read "Zoom time X"() -> (w468:bool)
              }
            }
            n326 = call-dynamic "SetFullSpeedTransfer.vi"("Full speed transfer"="High speed transfer to host", "ScopeBase In"=w454) -> ("ScopeBase Out"=w451:refnum<class "Scope5782_six_channel.lvclass">)  [unwired: 8 in, 1 out]
            n327 = property on="Zoom time X" class="Bool (strict)"("Val(Sgnl)"=w456) -> ()  [unwired: 2 in, 2 out]
          }
          event "Samples per 5782 record": Value Change {
            n328 = event-data() -> ()  [unwired: 1 in, 6 out]
            n329 = call-dynamic "SetRecordLength.vi"("Samples per 5782 record"="Samples per 5782 record", "ScopeBase In"=w472) -> ("ScopeBase Out"=w470:refnum<class "Scope5782_six_channel.lvclass">)  [unwired: 8 in, 1 out]
          }
          event "Singleshot": Value Change {
            n330 = event-data() -> ()  [unwired: 1 in, 6 out]
            n331 = local write "Rumode"(FALSE ("Rumode")) -> ()
            n332 = call-dynamic "SetRunMode.vi"("RunMode"=ScopeMode."Single" ("scope mode"), "ScopeBase in"=w473) -> ("ScopeBase out"=w474:refnum<class "Scope5782_six_channel.lvclass">)  [unwired: 8 in, 1 out]
          }
          event "Rumode": Value Change {
            n333 = event-data() -> ()  [unwired: 1 in, 6 out]
            n334 = case shown="\"Triggered\"" "Trigmode" {
              tunnel: [ScopeMode."Running" ("scope mode") ScopeMode."Continuous" ("scope mode")] -> w480
              frame "Triggered" {
              }
              frame "Continuous" {
              }
            }
            n335 = Select(t=w480, s="Rumode", f=ScopeMode."Stopped" ("scope mode")) -> (s? t:f=w479:T23)
            n336 = call-dynamic "SetRunMode.vi"("RunMode"=w479, "ScopeBase in"=w478) -> ("ScopeBase out"=w477:refnum<class "Scope5782_six_channel.lvclass">)  [unwired: 8 in, 1 out]
          }
          event "Unwrap phase": Value Change {
            w486 = dbl[][] [] ("History Data")
            n337 = event-data() -> ()  [unwired: 1 in, 6 out]
            n338 = property on="Lower chart" class="WFChart (strict)"("History Data"=w486) -> ()  [unwired: 2 in, 2 out]
            n339 = property on="Upper chart" class="WFChart (strict)"("History Data"=w486) -> ()  [unwired: 2 in, 2 out]
          }
          event "stop": Value Change {
            n340 = event-data() -> ()  [unwired: 1 in, 6 out]
          }
          event Value Change {
            n341 = event-data() -> ()  [unwired: 1 in, 6 out]
            n342 = case shown="\"V\"" "Unit" {
              tunnel: ["V" "dBV" "V^2"] -> w492
              frame "V" {
              }
              frame "dBV" {
              }
              frame "V^2" {
              }
            }
            n343 = Concatenate Strings("Amplitude [", w492, "]") -> (w490:string)
            n344 = property on="freqdata" class="WFGraph (strict)"("YScale.NameLbl.Text"=w490) -> ()  [unwired: 2 in, 2 out]
          }
          event "#bins": Value Change {
            n345 = event-data() -> ()  [unwired: 1 in, 6 out]
            n346 = local read "Upper chart"() -> (w502:dbl[][])
            n347 = local read "Window"() -> (w503:T8)
            n348 = local read "Unit"() -> (w504:T7)
            n349 = call "calc FFT_indexed.vi"("#bins"="#bins", "IQ indexes"=i32[][] [[0, 1], [2, 3], [4, 5], [6, 7], [8, 9], [10, 11], [12, 13]], "dt"=1e-06, "Unit"=w504, "Window"=w503, "data"=w502) -> ("Power Spectrum / PSD"=w501:cluster{"f0":dbl, "df":dbl, "magnitude":dbl[]}[])  [unwired: 5 in]
            n350 = local write "freqdata"(w501) -> ()
          }
          event "Zoom time X", "Zoom time Y": Value Change {
            n351 = event-data() -> ()  [unwired: 1 in, 6 out]
            n352 = control-ref of="Upper chart"() -> (w509:refnum<vi>)
            n353 = control-ref of="Upper graph"() -> (w510:refnum<vi>)
            n354 = call "setZoomTool.vi"("Zoom Y"="Zoom time Y", "Zoom  X"="Zoom time X", "reference"=w509) -> ()  [unwired: 9 in]
            n355 = call "setZoomTool.vi"("Zoom Y"="Zoom time Y", "Zoom  X"="Zoom time X", "reference"=w510) -> ()  [unwired: 9 in]
          }
          event "Zoom freq Y", "Zoom freq X": Value Change {
            n356 = event-data() -> ()  [unwired: 1 in, 6 out]
            n357 = control-ref of="Lower chart"() -> (w516:refnum<vi>)
            n358 = control-ref of="Lower graph"() -> (w515:refnum<vi>)
            n359 = control-ref of="Adaptive FF graph"() -> (w512:refnum<vi>)
            n360 = control-ref of="freqdata"() -> (w517:refnum<vi>)
            n361 = call "setZoomTool.vi"("Zoom Y"="Zoom freq Y", "Zoom  X"="Zoom freq X", "reference"=w517) -> ()  [unwired: 9 in]
            n362 = call "setZoomTool.vi"("Zoom Y"="Zoom freq Y", "Zoom  X"="Zoom freq X", "reference"=w512) -> ()  [unwired: 9 in]
            n363 = call "setZoomTool.vi"("Zoom Y"="Zoom freq Y", "Zoom  X"="Zoom freq X", "reference"=w516) -> ()  [unwired: 9 in]
            n364 = call "setZoomTool.vi"("Zoom Y"="Zoom freq Y", "Zoom  X"="Zoom freq X", "reference"=w515) -> ()  [unwired: 9 in]
          }
          event "Show buffers": Value Change {
            n365 = event-data() -> ("CtlRef"=w521:refnum<vi>)  [unwired: 1 in, 5 out]
            n366 = control-ref of="Show buffers"() -> (w520:refnum<vi>)
            n367 = Equal?(x=w521, y=w520) -> (x = y?=w519:bool)
            n368 = case shown="False" w519 {
              frame False {
                w529 = dbl[][] [] ("History Data")
                n369 = local write "freqdata"(cluster{"f0":dbl, "df":dbl, "magnitude":dbl[]}[] [] ("freqdata")) -> ()
                n370 = property on="Upper chart" class="WFChart (strict)"("History Data"=w529) -> ()  [unwired: 2 in, 2 out]
                n371 = property on="Lower chart" class="WFChart (strict)"("History Data"=w529) -> ()  [unwired: 2 in, 2 out]
              }
              frame True {
              }
            }
            n372 = call "UpdateGraphs.vi"("Show buffers"="Show buffers", "Buffer mode"="Buffer", "Display mode"="Display", "Graph_refs"=w524) -> ()  [unwired: 8 in]
            n373 = property on="Zoom time X" class="Bool (strict)"("Val(Sgnl)"=TRUE ("Value (Signaling)")) -> ()  [unwired: 2 in, 2 out]
          }
          event "Feed forward": Value Change {
            n374 = event-data() -> ()  [unwired: 1 in, 6 out]
            n375 = control-ref of="show feedforward"() -> (w536:refnum<vi>)
            n376 = call "LoadFeedforward.vi"("show ref"=w536, "Path"="Feed forward") -> ("error out"=w531:errorcluster, "values Q"=w532:dbl[], "values I"=w533:dbl[])  [unwired: 7 in]
            n377 = call "SetFeedForward.vi"("error in (no error)"=w531, "values Q"=w532, "values I"=w533, "Scope5785_six_channel"=w534) -> ("Scope5785_six_channel out"=w530:refnum<class "Scope5782_six_channel.lvclass">)  [unwired: 6 in, 1 out]
          }
          event "Beam": Value Change {
            n378 = event-data() -> ()  [unwired: 1 in, 6 out]
            n379 = control-ref of="show beam"() -> (w542:refnum<vi>)
            n380 = call "LoadFeedforward.vi"("show ref"=w542, "Path"="Beam") -> ("error out"=w537:errorcluster, "values Q"=w538:dbl[], "values I"=w539:dbl[])  [unwired: 7 in]
            n381 = call "SetBeam.vi"("error in (no error)"=w537, "values Q"=w538, "values I"=w539, "Scope5785_six_channel"=w544) -> ("error out"=w541:errorcluster, "Scope5785_six_channel out"=w543:refnum<class "Scope5782_six_channel.lvclass">)  [unwired: 6 in]
            n382 = property class="Bool"(reference=w542, error in=w541, "DisabledEnum"=T24."Enabled" ("Disabled")) -> ()  [unwired: 2 out]
          }
          event "Setpoint": Value Change {
            n383 = event-data() -> ()  [unwired: 1 in, 6 out]
            n384 = control-ref of="show setpoint"() -> (w552:refnum<vi>)
            n385 = call "LoadFeedforward.vi"("show ref"=w552, "Path"="Setpoint") -> ("error out"=w547:errorcluster, "values Q"=w549:dbl[], "values I"=w550:dbl[])  [unwired: 7 in]
            n386 = call "SetSetpoint.vi"("error in (no error)"=w547, "values Q"=w549, "values I"=w550, "Scope5785_six_channel"=w548) -> ("Scope5785_six_channel out"=w546:refnum<class "Scope5782_six_channel.lvclass">)  [unwired: 6 in, 1 out]
          }
          event "Input delay 5761": Value Change {
            n387 = event-data() -> ()  [unwired: 1 in, 6 out]
            n388 = call "Read FpgaRef5761.vi"("Scope5785_six_channel"=w557) -> ("FpgaRef5761.lvclass"=w555:refnum<class "FpgaRef5761.lvclass">, "Scope5785_six_channel Out"=w556:refnum<class "Scope5782_six_channel.lvclass">)  [unwired: 8 in, 1 out]
            n389 = call "WriteSetting 32bit.vi"("value"="Input delay 5761", "FPGA Setting"=fpga_settings."Input delay", "FpgaRefBase in"=w555) -> ()  [unwired: 7 in, 2 out]
          }
          event "Input delay 5785": Value Change {
            n390 = event-data() -> ()  [unwired: 1 in, 6 out]
            n391 = call "Read FpgaRef5782.vi"("Scope5785_six_channel"=w562) -> ("FpgaRef5782.lvclass"=w560:refnum<class "FpgaRef5782.lvclass">, "Scope5785_six_channel Out"=w561:refnum<class "Scope5782_six_channel.lvclass">)  [unwired: 8 in, 1 out]
            n392 = call "WriteSetting 32bit.vi"("value"="Input delay 5785", "FPGA Setting"=fpga_settings."Input delay", "FpgaRefBase in"=w560) -> ()  [unwired: 7 in, 2 out]
          }
          event Value Change {
            n393 = event-data() -> ()  [unwired: 1 in, 6 out]
            n394 = call "Read FpgaRef5782.vi"("Scope5785_six_channel"=w567) -> ("FpgaRef5782.lvclass"=w565:refnum<class "FpgaRef5782.lvclass">, "Scope5785_six_channel Out"=w566:refnum<class "Scope5782_six_channel.lvclass">)  [unwired: 8 in, 1 out]
            n395 = call "WriteSetting 16bit.vi"("value"="Output scale", "FPGA Setting"=fpga_settings."Output scale", "FpgaRefBase in"=w565) -> ()  [unwired: 7 in, 2 out]
          }
          event Value Change {
            n396 = event-data() -> ()  [unwired: 1 in, 6 out]
            n397 = call "Read FpgaRef5782.vi"("Scope5785_six_channel"=w572) -> ("FpgaRef5782.lvclass"=w570:refnum<class "FpgaRef5782.lvclass">, "Scope5785_six_channel Out"=w571:refnum<class "Scope5782_six_channel.lvclass">)  [unwired: 8 in, 1 out]
            n398 = call "WriteSetting 16bit.vi"("value"="Input scale", "FPGA Setting"=fpga_settings."Input scale", "FpgaRefBase in"=w570) -> ()  [unwired: 7 in, 2 out]
          }
          event Value Change {
            n399 = event-data() -> ()  [unwired: 1 in, 6 out]
            n400 = call "Read FpgaRef5761.vi"("Scope5785_six_channel"=w575) -> ("FpgaRef5761.lvclass"=w573:refnum<class "FpgaRef5761.lvclass">, "Scope5785_six_channel Out"=w574:refnum<class "Scope5782_six_channel.lvclass">)  [unwired: 8 in, 1 out]
            n401 = call "WriteSetting 16bit.vi"("value"="Input scale 5761", "FPGA Setting"=fpga_settings."Input scale", "FpgaRefBase in"=w573) -> ()  [unwired: 7 in, 2 out]
          }
          event Value Change {
            n402 = event-data() -> ()  [unwired: 1 in, 6 out]
            n403 = call "Read FpgaRef5761.vi"("Scope5785_six_channel"=w581) -> ("FpgaRef5761.lvclass"=w579:refnum<class "FpgaRef5761.lvclass">, "Scope5785_six_channel Out"=w580:refnum<class "Scope5782_six_channel.lvclass">)  [unwired: 8 in, 1 out]
            n404 = call "WriteSetting 16bit.vi"("value"="Host scale 5761", "FPGA Setting"=fpga_settings."Host scale", "FpgaRefBase in"=w579) -> ()  [unwired: 7 in, 2 out]
          }
          event Value Change {
            n405 = event-data() -> ()  [unwired: 1 in, 6 out]
            n406 = call "Read FpgaRef5782.vi"("Scope5785_six_channel"=w587) -> ("FpgaRef5782.lvclass"=w585:refnum<class "FpgaRef5782.lvclass">, "Scope5785_six_channel Out"=w586:refnum<class "Scope5782_six_channel.lvclass">)  [unwired: 8 in, 1 out]
            n407 = call "WriteSetting 16bit.vi"("value"="Host scale", "FPGA Setting"=fpga_settings."Host scale", "FpgaRefBase in"=w585) -> ()  [unwired: 7 in, 2 out]
          }
          event "Adaptive FF enabled", "LP filter cutoff fequency [MHz]", "Adaptation factor [0-1]", "Samples to skip": Value Change {
            n408 = event-data() -> ()  [unwired: 1 in, 6 out]
            n409 = call "Read FpgaRef5782.vi"("Scope5785_six_channel"=w594) -> ("FpgaRef5782.lvclass"=w592:refnum<class "FpgaRef5782.lvclass">, "Scope5785_six_channel Out"=w593:refnum<class "Scope5782_six_channel.lvclass">)  [unwired: 8 in, 1 out]
            n410 = call "Write Adaptive FF settings.vi"("Samples to skip"="Samples to skip", "Adaptation factor [0-1]"="Adaptation factor [0-1]", "LP filter cutoff fequency [MHz]"="LP filter cutoff fequency [MHz]", "Adaptive FF enabled"="Adaptive FF enabled", "FpgaRef5785 in"=w592) -> ()  [unwired: 6 in, 1 out]
          }
          event "IIR filter cutoff fequency [MHz]": Value Change {
            n411 = event-data() -> ()  [unwired: 1 in, 6 out]
            n412 = call "Read FpgaRef5782.vi"("Scope5785_six_channel"=w599) -> ("FpgaRef5782.lvclass"=w597:refnum<class "FpgaRef5782.lvclass">, "Scope5785_six_channel Out"=w598:refnum<class "Scope5782_six_channel.lvclass">)  [unwired: 8 in, 1 out]
            n413 = call "Write Adaptive FF IIR coeffs.vi"("Fs [MHz}"=10.0, "cutoff fequency [MHz]"="IIR filter cutoff fequency [MHz]", "FpgaRef5785 in"=w597) -> ()  [unwired: 8 in, 1 out]
          }
          event "Read buffers": Value Change {
            n414 = event-data() -> ()  [unwired: 1 in, 6 out]
            n415 = call "Read Trigger.vi"("ScopeBase in"=w605) -> ("5782 trigger"=w603:T5, "ScopeBase out"=w604:refnum<class "Scope5782_six_channel.lvclass">)  [unwired: 8 in, 1 out]
            n416 = call "Read scope mode.vi"("ScopeBase in"=w604) -> ("scope mode"=w608:T23, "ScopeBase out"=w609:refnum<class "Scope5782_six_channel.lvclass">)  [unwired: 8 in, 1 out]
            n417 = call "Read FpgaRef5782.vi"("Scope5785_six_channel"=w609) -> ("FpgaRef5782.lvclass"=w612:refnum<class "FpgaRef5782.lvclass">, "Scope5785_six_channel Out"=w613:refnum<class "Scope5782_six_channel.lvclass">)  [unwired: 8 in, 1 out]
            n418 = Equal?(x=w603, y=5782_trigger_type."Software") -> (x = y?=w601:bool)
            n419 = Not Equal?(x=w608, y=ScopeMode."Running") -> (x != y?=w606:bool)
            n420 = Or(x=w606, y=w601) -> (x .or. y?=w600:bool)
            n421 = call "Read FF buffers.vi"("Force"=w600, "FpgaRef5785 in"=w612) -> ("Scaled"=w611:dbl[][])  [unwired: 7 in, 2 out]
            n422 = flat-sequence {
              tunnel: w611 -> [w614]
              frame #0 {
                "Adaptive FF graph" <- w614
              }
            }
            n423 = property on="Show buffers" class="Bool (strict)"("Val(Sgnl)"=TRUE ("Value (Signaling)")) -> ()  [unwired: 2 in, 2 out]
          }
          event "Save FF to file": Value Change {
            n424 = event-data() -> ()  [unwired: 1 in, 6 out]
            n425 = call "File Dialog"("prompt"="Select file", "pattern (all files)"="*.txt", "pattern label"="Text file") -> ("selected path"=w615:path, "error out"=w616:errorcluster)  [unwired: 9 in, 2 out]
            n426 = case shown="No Error" w616 {
              tunnel: w615 -> [w624 _]
              frame No Error {
                n427 = local read "Adaptive FF graph"() -> (w621:dbl[][])
                n428 = Index Array(array=w621, index (row) #1=2 ("index (row)"), index (row) #2=3 ("index (row)")) -> (element #1=w623:dbl[], element #2=w622:dbl[])  [unwired: 2 in]
                n429 = call "SaveFeedForwardFile.vi"("values Q"=w622, "values I"=w623, "Path"=w624) -> ()  [unwired: 8 in, 1 out]
              }
              frame Error {
              }
            }
          }
          event "Clear buffers": Value Change {
            n430 = event-data() -> ()  [unwired: 1 in, 6 out]
            n431 = call "Read Trigger.vi"("ScopeBase in"=w630) -> ("5782 trigger"=w633:T5, "ScopeBase out"=w627:refnum<class "Scope5782_six_channel.lvclass">)  [unwired: 8 in, 1 out]
            n432 = call "Read scope mode.vi"("ScopeBase in"=w627) -> ("scope mode"=w636:T23, "ScopeBase out"=w635:refnum<class "Scope5782_six_channel.lvclass">)  [unwired: 8 in, 1 out]
            n433 = call "Read FpgaRef5782.vi"("Scope5785_six_channel"=w635) -> ("FpgaRef5782.lvclass"=w637:refnum<class "FpgaRef5782.lvclass">, "Scope5785_six_channel Out"=w638:refnum<class "Scope5782_six_channel.lvclass">)  [unwired: 8 in, 1 out]
            n434 = Not Equal?(x=w636, y=ScopeMode."Running") -> (x != y?=w629:bool)
            n435 = Equal?(x=w633, y=5782_trigger_type."Software") -> (x = y?=w631:bool)
            n436 = Or(x=w629, y=w631) -> (x .or. y?=w628:bool)
            n437 = call "Clear FF buffers.vi"("Force"=w628, "FpgaRef5785 in"=w637) -> ()  [unwired: 8 in, 2 out]
          }
        }
        n438 = case shown="False" w155 {
          tunnel: w154 -> [w165 _]
          frame False {
            n439 = Generate User Event(user event=w165, event data cluster=T21 {"Automatic"=TRUE, "Save"=TRUE} ("event data")) -> ()  [unwired: 2 in, 2 out]
          }
          frame True {
          }
        }
      }
      "stop 2" <- w148
    }
    frame Error {
    }
  }
  n440 = call "Run.vi"("SettingsFile in"=w11) -> ()  [unwired: 10 in, 1 out]
  n441 = Unregister For Events(event registration refnum=w99) -> ()  [unwired: 1 in, 1 out]
  n442 = call-dynamic "Close.vi"("ScopeBase in"=w66) -> ("error out"=w65:errorcluster)  [unwired: 10 in]
  n443 = flat-sequence {
    tunnel: w65 -> [_]
    frame #0 {
      n444 = global write "global_stop.vi" "Stop"(TRUE ("Stop")) -> ()
    }
  }
